vi "Hardware - XNET CAN Host.vi"() -> ()   [LabVIEW 2015, in "ECS-Host.lvlib"]
uses:
  ECS-Host.lvlib
  Typedefs/MISC/Control Parameters.ctl
  ECS-Shared.lvlib
panel:
  out "Loop Duration":u32 caption="[ms]"
  in  "Loop Period":u32 caption="[ms]"
  in  "Refresh Database":bool
  out "CAN Tx Signals":sgl[](array[numeric])
  out "Tx Data":sgl[](array[numeric]) caption="data" format="%.2f"
  in  "Tx Signals":string
  in  "_Tx Signals Mem":string[](array[string])
  in  "CalPointIDs":sgl[](array[numeric])
  out "NamesShort":string
  out "CAN Rx Signals":sgl[](array[numeric])
  in  "Rx Signals":string
  out "Rx Data":sgl[](array[numeric]) caption="data" format="%.2f"
  in  "_Rx Signals Mem":string[](array[string])
  in  "ControlParamMem":string
  in  "_Control Param Array":T1[](array[typedef])
  out "XNET_Fault":bool
  in  "_Refresh (Hidden)":bool
  out "DatabaseAlias":string
  out "CAN Interfaces":sgl[](array[numeric])
  out "IP_Address":string="0.0.0.0"
  in  "CAN Interface":u8
  out "CAN ECUs":sgl[](array[numeric])
  out "CAN Clusters":sgl[](array[numeric])
  out "XNET_Fault_Code":i32
  out "XNET_Fault_Desc":string
  in  "_CalPoints Select":u32(ring) caption="CalPoints Select"
  out "_XNET Error":T2 caption="XNET Error"
  in  "Deployed ECUs":i32(listbox) caption="Deployed Databases"
  in  "Deployed Clusters":i32(listbox) caption="Deployed Databases"
  in  "Intf_CAN_Term":bool caption="Termination"
  in  "Baud_Rate":u32 caption="Baud Rate"
  in  "Deployed Databases":i32(listbox)
  in  "CAN_Run":bool
  in  "_CAN Tx Signal":u16(ring) caption="CAN Signal" items=["Not Selected"]
  in  "_Tx.Insert":bool
  in  "_Tx.Up":bool
  in  "_Tx.Delete":bool
  in  "_Tx.Down":bool
  in  "_Tx Table":i32(listbox)
  in  "_CAN Rx Signal":u16(ring) caption="CAN Signal" items=["Not Selected"]
  in  "_Rx.Insert":bool
  in  "_Rx.Up":bool
  in  "_Rx.Delete":bool
  in  "_Rx.Down":bool
  in  "_CAN Interface":u8(ring) caption="CAN Interface"
  in  "_Control Parameter":T1=enum."Pedal Position [%]" caption="Control Parameters"
  in  "_Rx Table":i32(listbox)
  # "---- Rx ---->"
  # "READ FROM\nCAN BUS"
  # "-------- Tx -------->"
  # "WRITE TO\nCAN BUS"
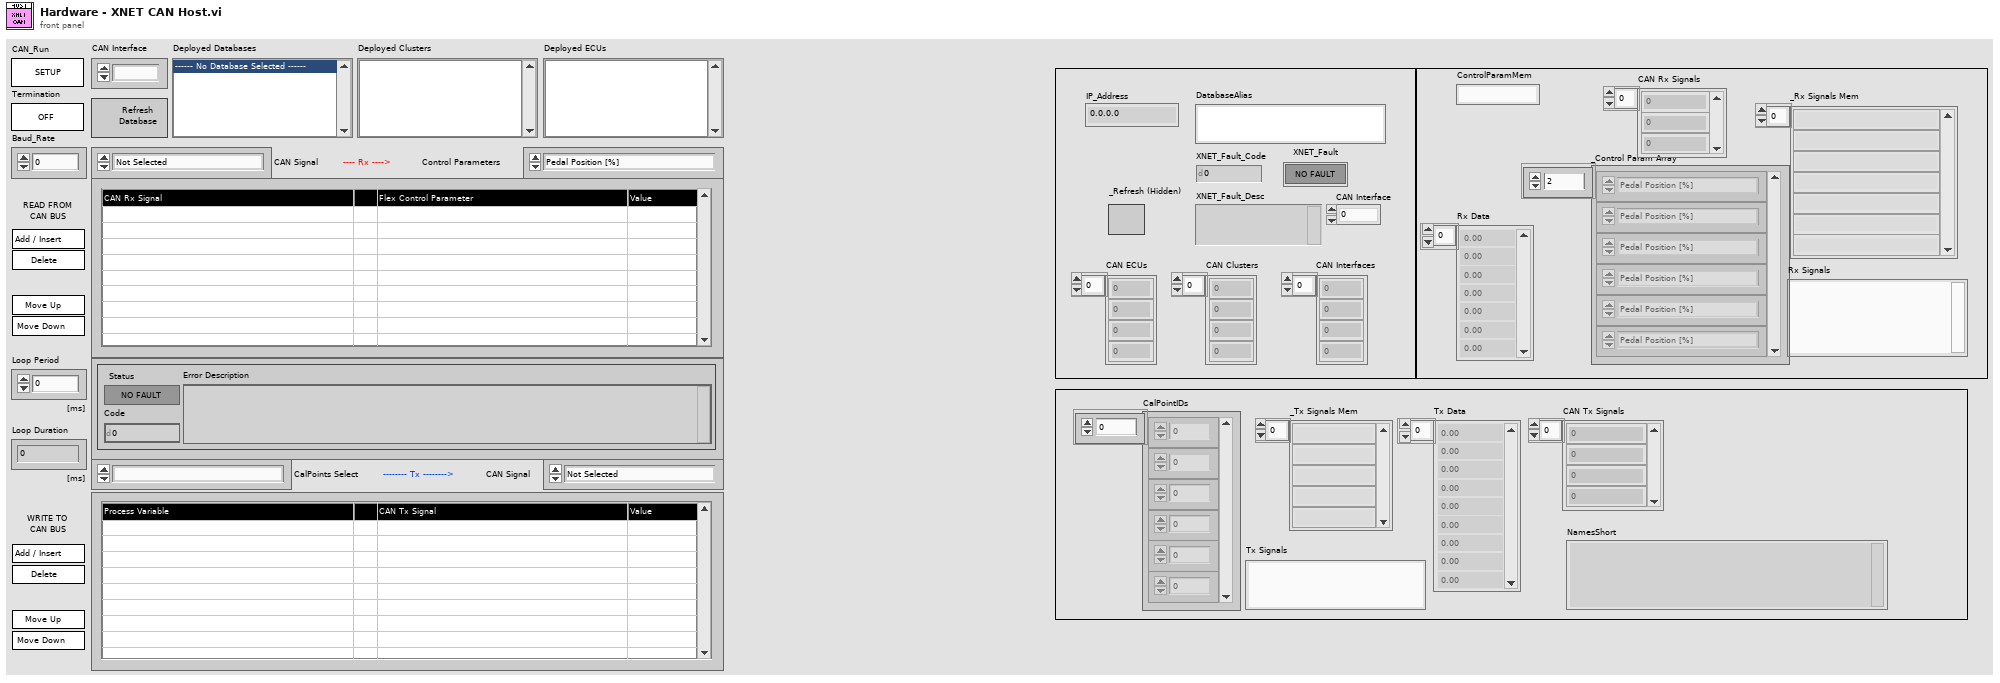
[diagram p1: front panel]
types:
  T1 = typedef "ECS-Shared.lvlib/Control Parameters.ctl" = enum16{"Not Selected", "Pedal Position [%]", "ESTOP", "Sensor1NOx", "Sensor1O2", "Sensor1SupplyStatus", "Sensor1TempStatus", "Sensor1NOxStatus", "Sensor1O2Status", "Sensor1HeaterMode", "Sensor1HeaterCircuit", "Sensor1NOxCircuit", "Sensor1O2Circuit", "Sensor2NOx", "Sensor2O2", "Sensor2SupplyStatus", "Sensor2TempStatus", "Sensor2NOxStatus", "Sensor2O2Status", "Sensor2HeaterMode", "Sensor2HeaterCircuit", "Sensor2NOxCircuit", "Sensor2O2Circuit"}
  T2 = cluster{"Status":bool, "Code":i32, "Error Description":string}
  T3 = enum8{"Enabled", "Disabled", "Disabled and Grayed Out"}
  T4 = cluster{"Status":bool, "Code":i32, "Desc":string}
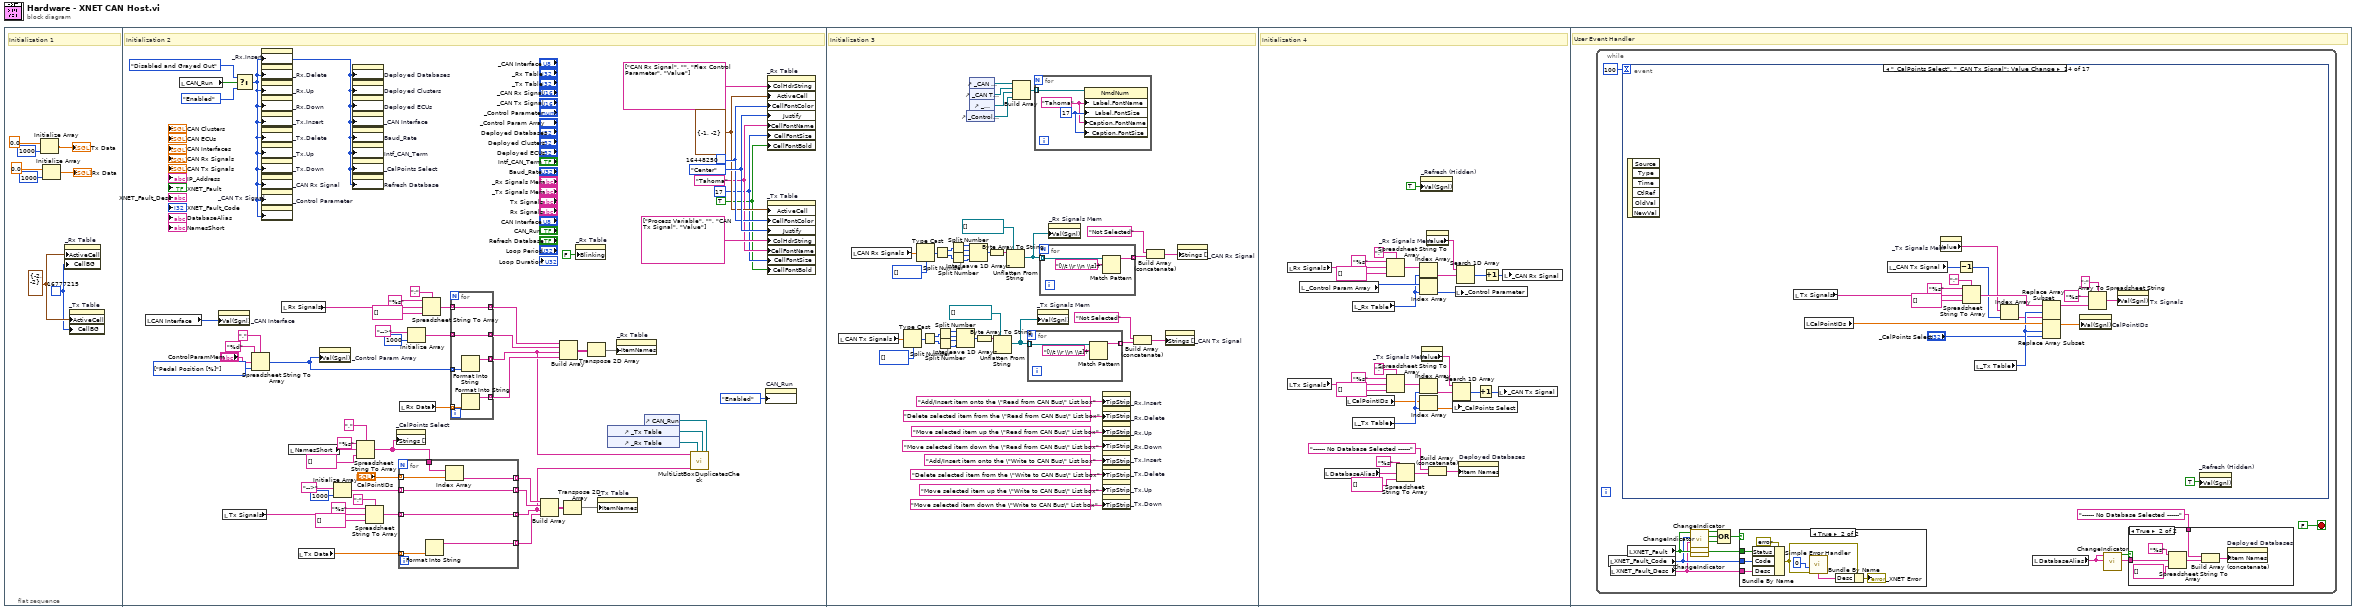
[diagram p0: block diagram]
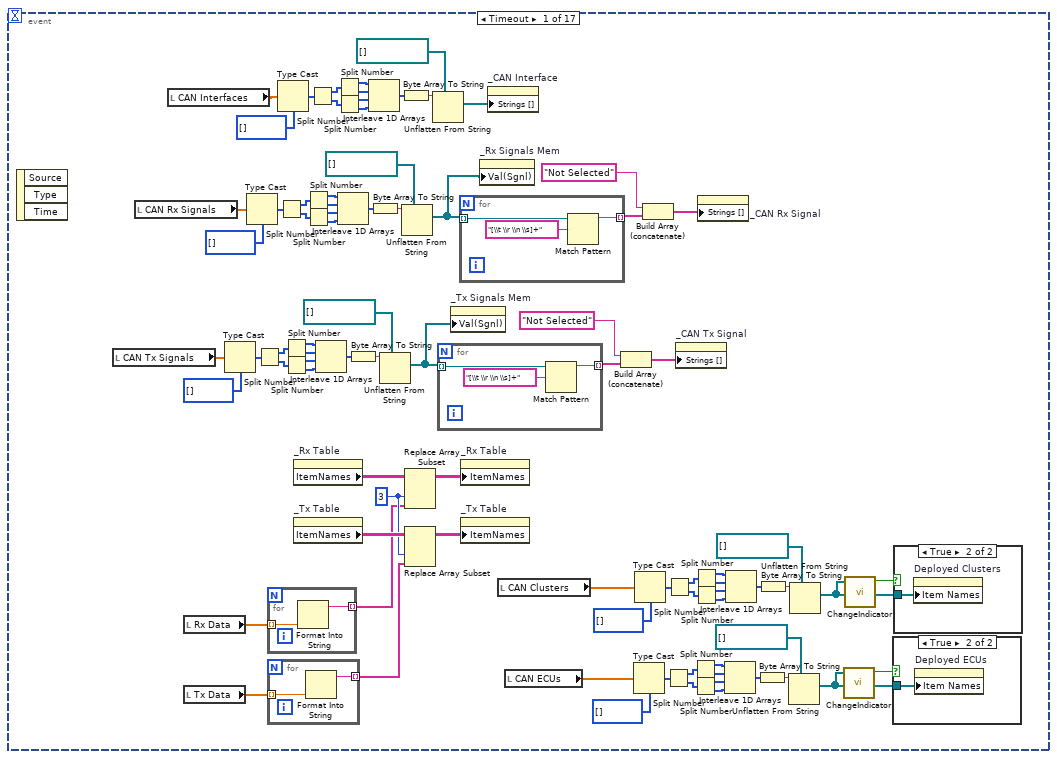
[diagram p4: hidden frame]
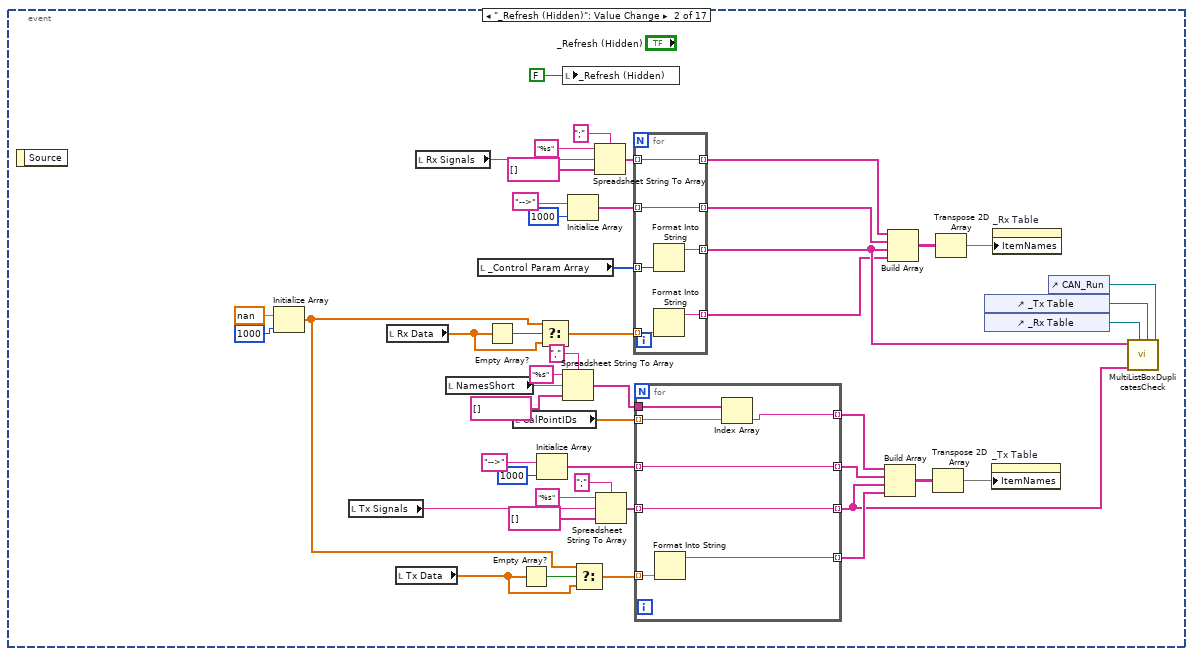
[diagram p7: hidden frame]
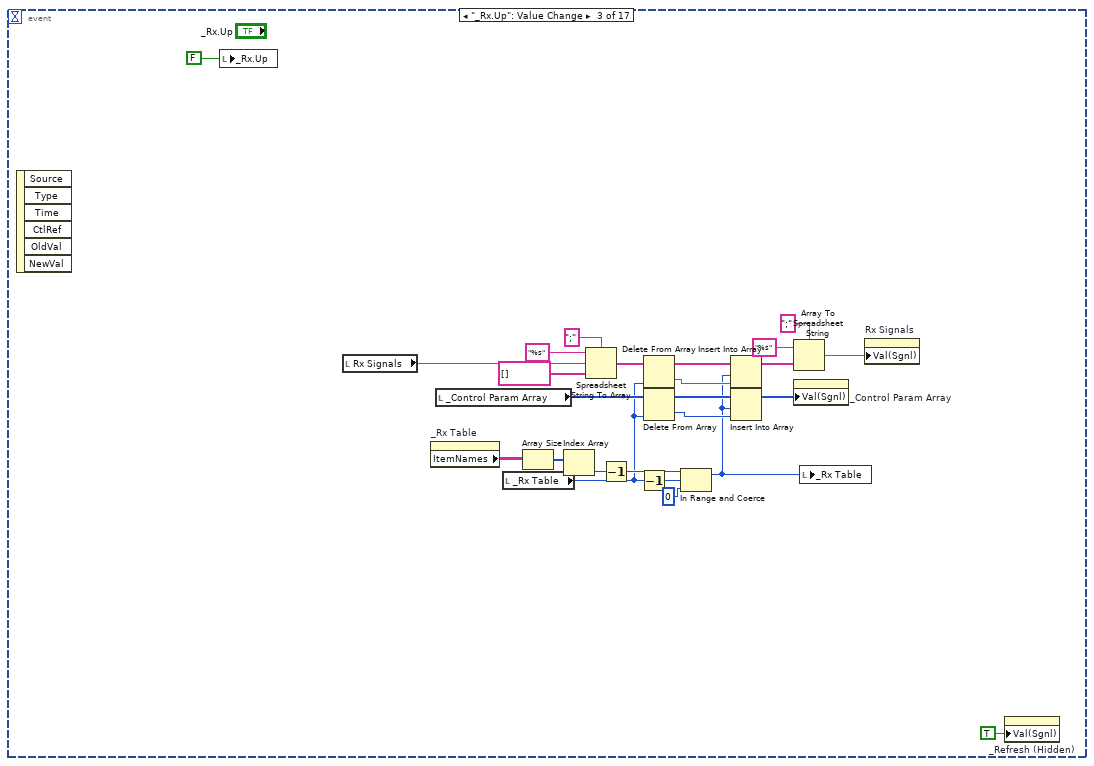
[diagram p8: hidden frame]
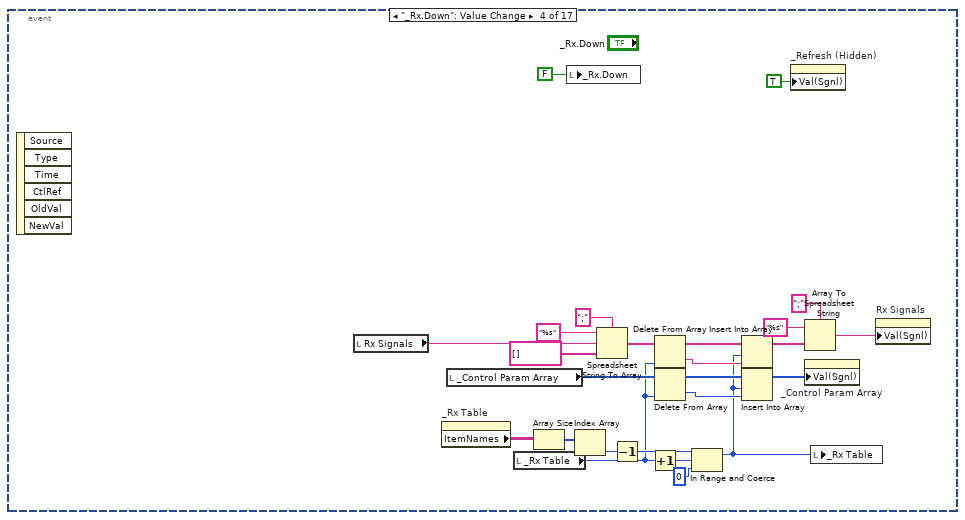
[diagram p9: hidden frame]
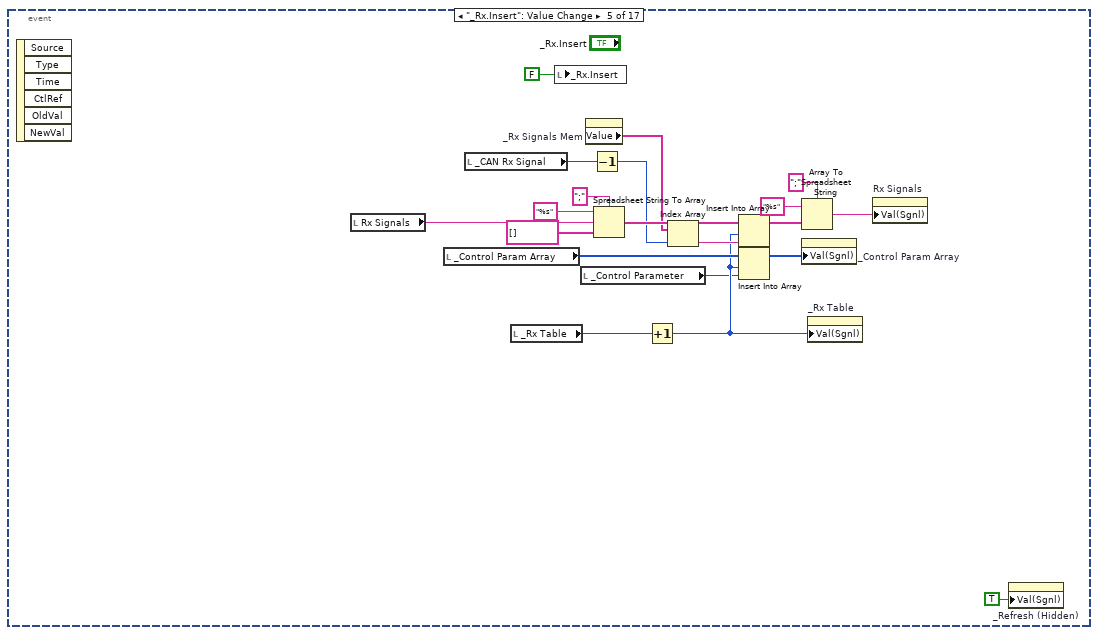
[diagram p10: hidden frame]
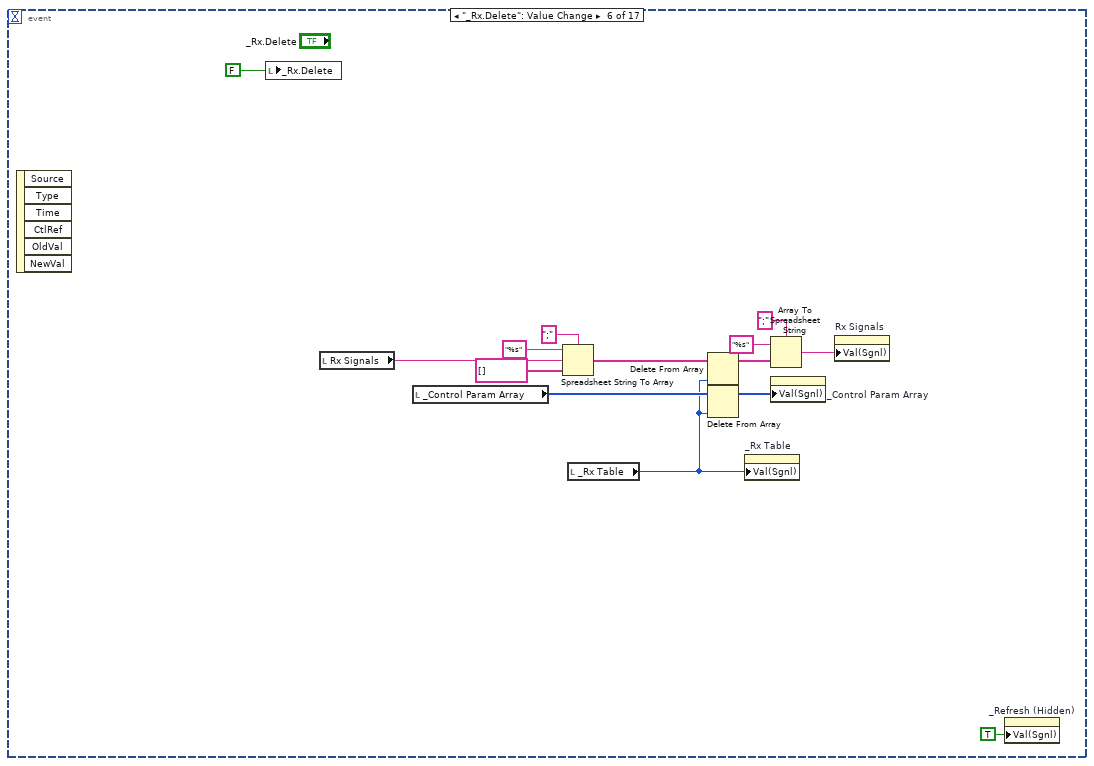
[diagram p11: hidden frame]
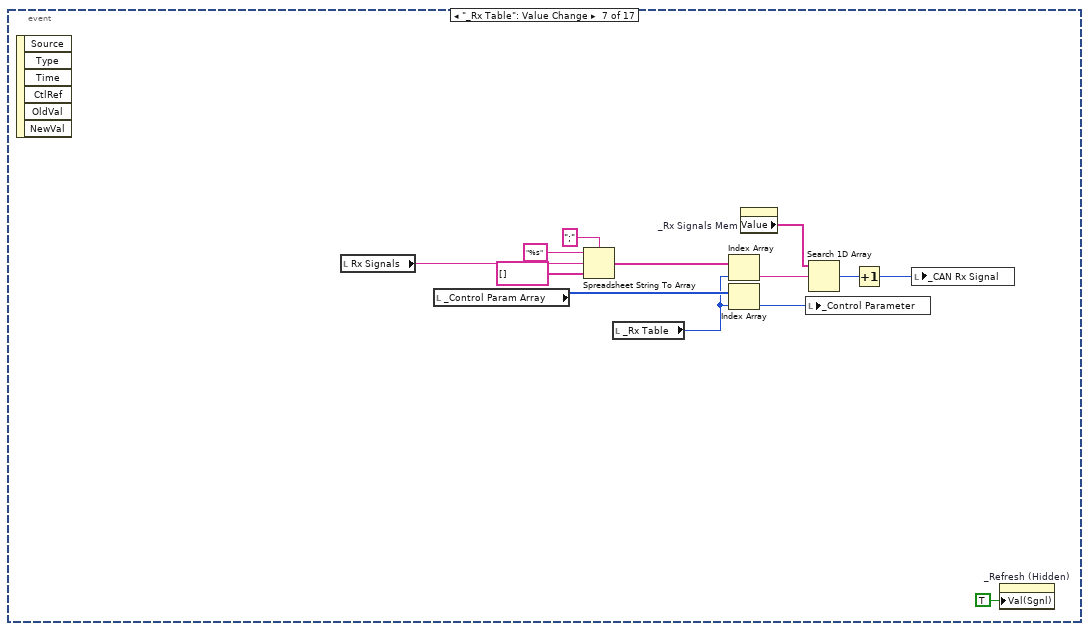
[diagram p12: hidden frame]
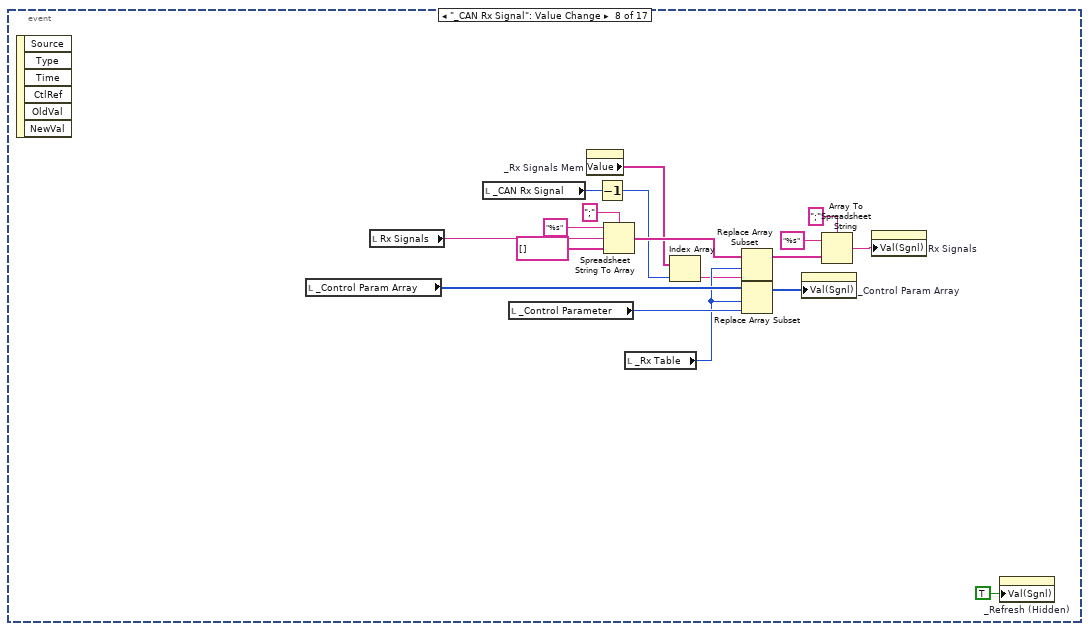
[diagram p13: hidden frame]
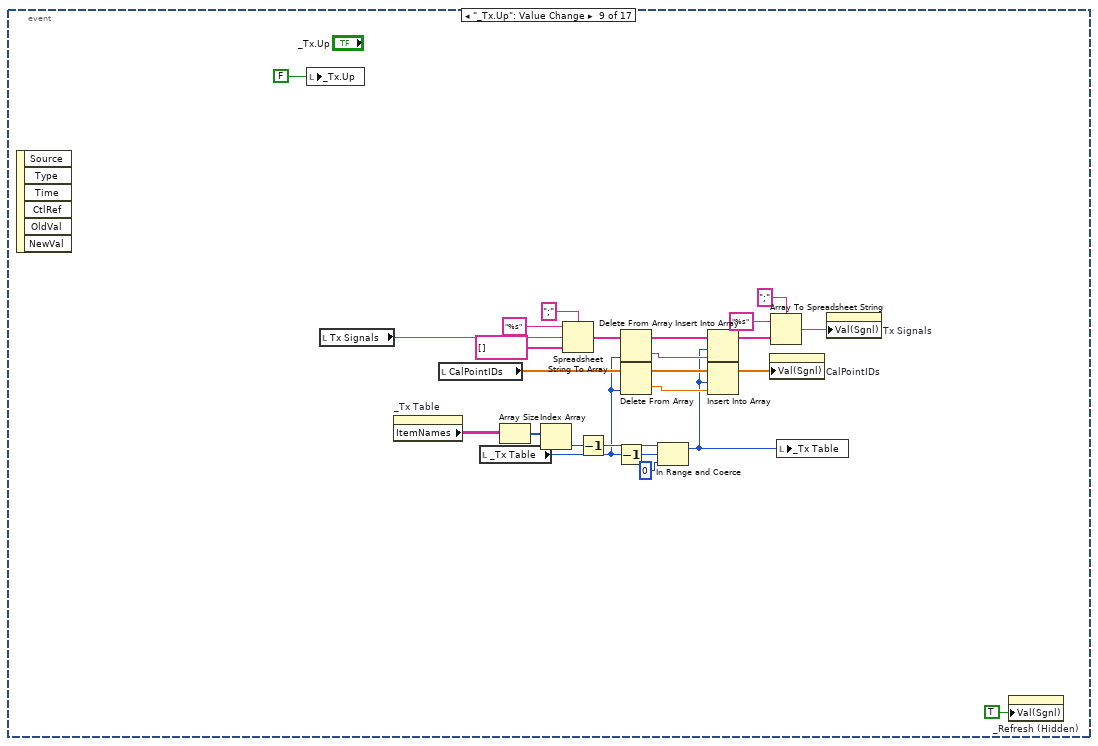
[diagram p14: hidden frame]
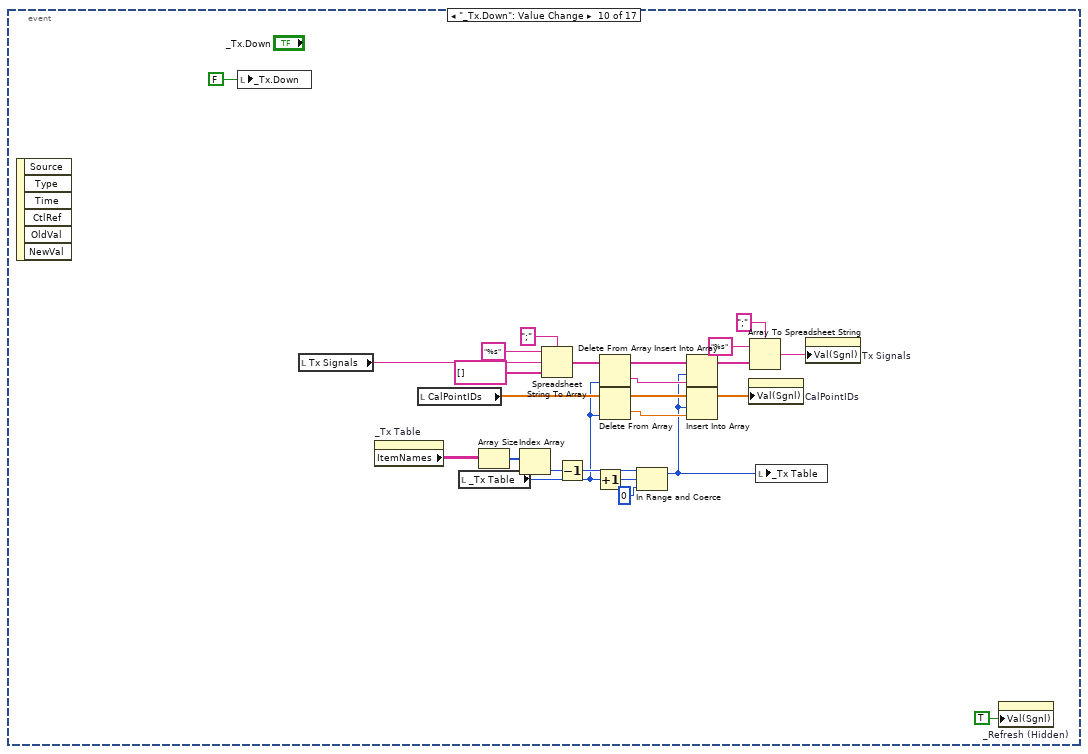
[diagram p15: hidden frame]
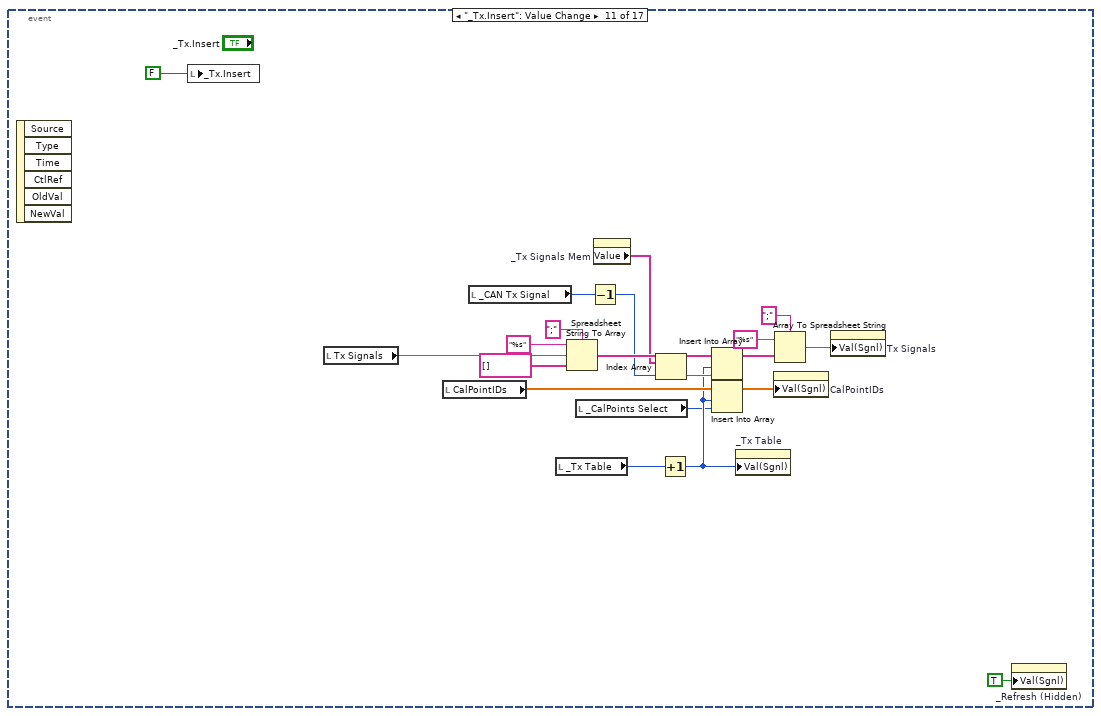
[diagram p16: hidden frame]
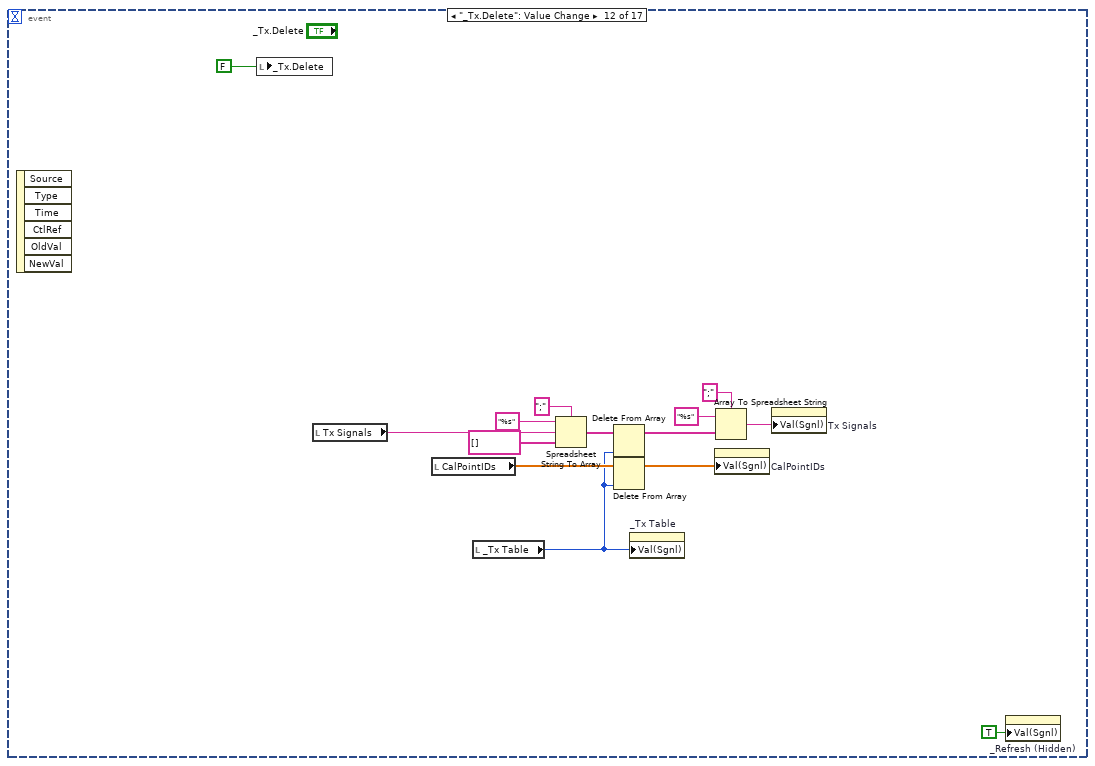
[diagram p17: hidden frame]
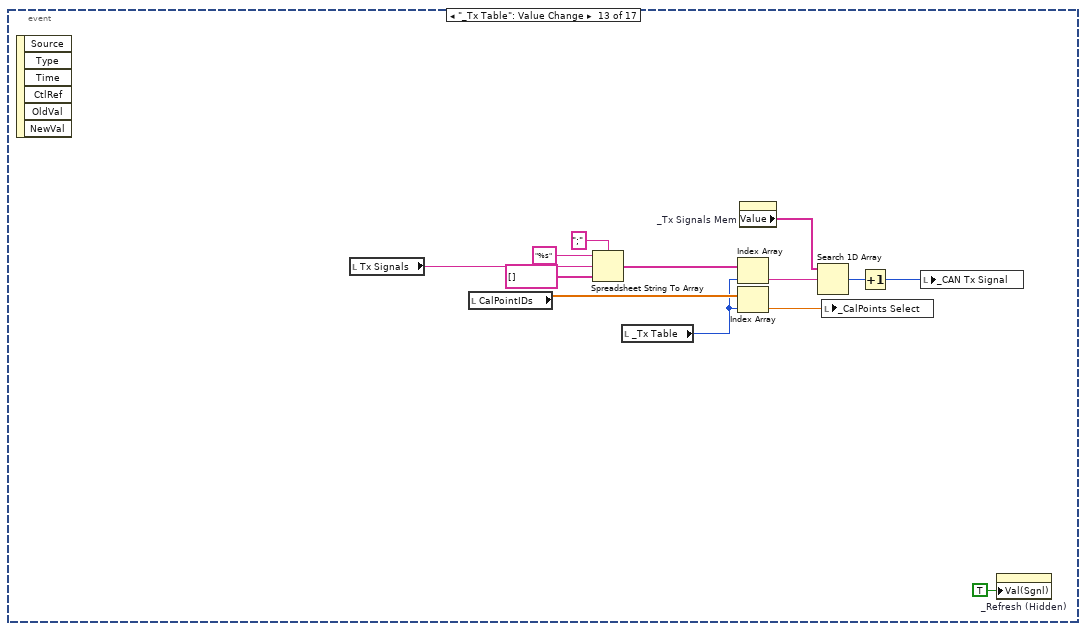
[diagram p18: hidden frame]
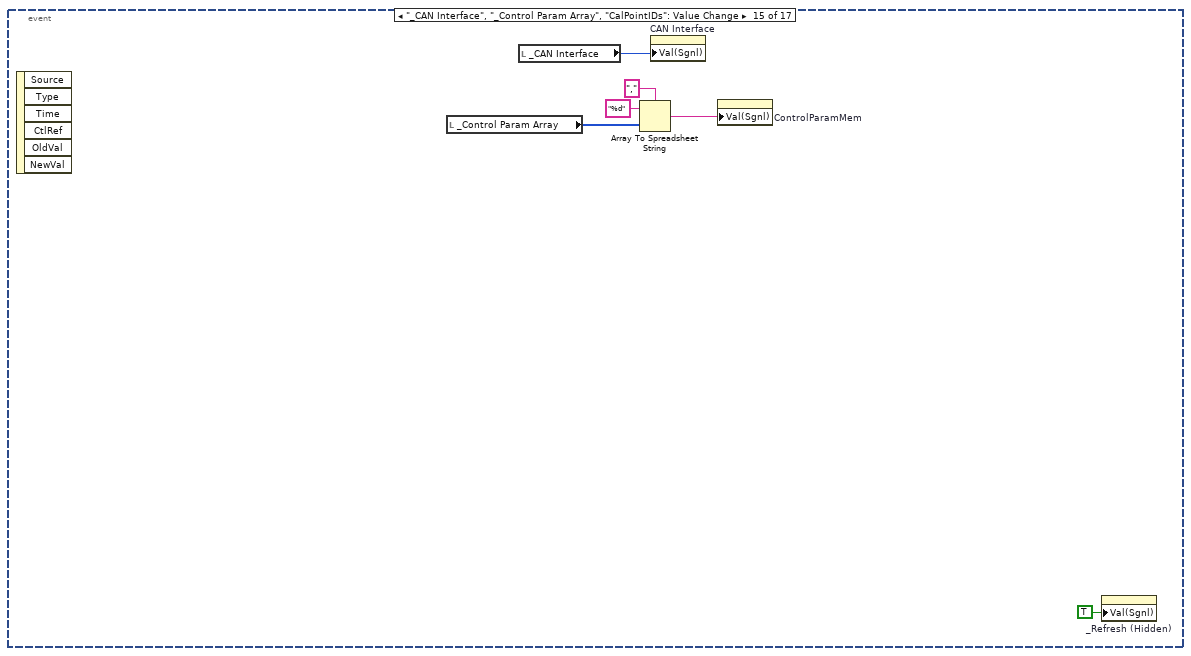
[diagram p19: hidden frame]
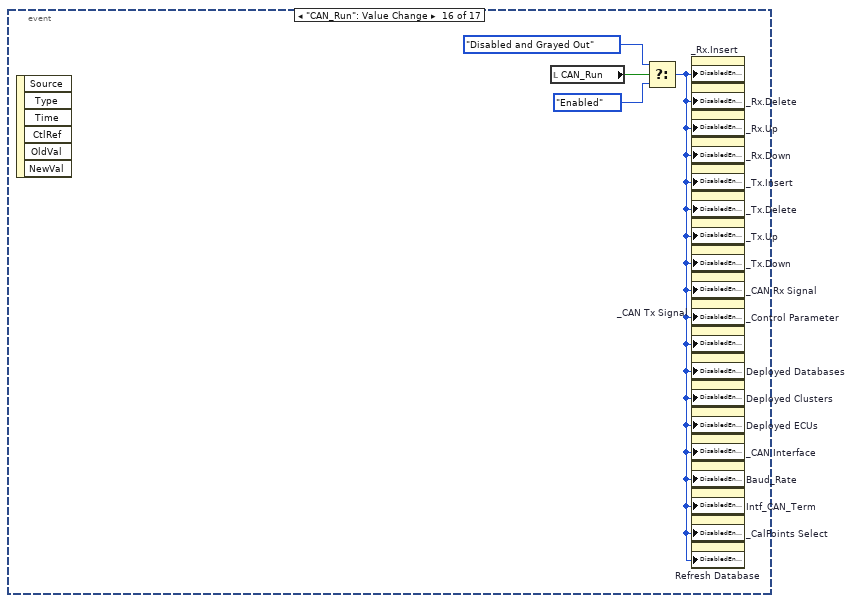
[diagram p20: hidden frame]
diagram:
  n1 = flat-sequence {
    frame #0 {
      w8 = cluster{"Row":i32, "Column":i32} {"Row"=-2, "Column"=-2} ("Active Cell:Active Cell")
      w7 = u32 16777215 ("Color Box")
      # "Initialization 1"
      n2 = Initialize Array(0.0, 1000 ("dimension size")) -> (→"Tx Data":dbl[])
      n3 = Initialize Array(0.0, 1000 ("dimension size")) -> (→"Rx Data":dbl[])
      n4 = property on="_Rx Table" class="MCListbox (strict)"("ActiveCell"=w8, "CellBG"=w7) -> ()  [unwired: 2 in, 2 out]
      n5 = property on="_Tx Table" class="MCListbox (strict)"("ActiveCell"=w8, "CellBG"=w7) -> ()  [unwired: 2 in, 2 out]
    }
    frame #1 {
      w24 = TRUE ("Active Cell:Cell Font:Bold")
      w25 = u32 17 ("Active Cell:Cell Font:Size")
      w26 = "Tahoma" ("Active Cell:Cell Font:Name")
      w29 = enum16{"Left", "Center", "Right"}."Center" ("Active Cell:Cell Justification")
      w28 = u32 16448250
      w27 = cluster{"Row":i32, "Column":i32} {"Row"=-1, "Column"=-2} ("Active Cell:Active Cell")
      w33 = T1[] [enum."Pedal Position [%]"] items=["Not Selected", "Pedal Position [%]", "ESTOP", "Sensor1NOx", "Sensor1O2", "Sensor1SupplyStatus", "Sensor1TempStatus", "Sensor1NOxStatus", "Sensor1O2Status", "Sensor1HeaterMode", "Sensor1HeaterCircuit", "Sensor1NOxCircuit", "Sensor1O2Circuit", "Sensor2NOx", "Sensor2O2", "Sensor2SupplyStatus", "Sensor2TempStatus", "Sensor2NOxStatus", "Sensor2O2Status", "Sensor2HeaterMode", "Sensor2HeaterCircuit", "Sensor2NOxCircuit", "Sensor2O2Circuit"]
      # "Initialization 2"
      n6 = local read "CAN Interface"() -> (w38:u8)
      n7 = local read "CAN_Run"() -> (w35:bool)
      n8 = property on="_CAN Interface" class="Ring (strict)"("Val(Sgnl)"=w38) -> ()  [unwired: 2 in, 2 out]
      n9 = local read "Tx Signals"() -> (w65:string)
      n10 = Select(t=T3."Disabled and Grayed Out" ("Disabled"), s=w35, f=T3."Enabled" ("Disabled")) -> (s? t:f=w9:T3)
      n11 = Spreadsheet String To Array(delimiter (Tab)=",", format string="%d", spreadsheet string="ControlParamMem", array type (2D Dbl)=w33) -> (array=w31:T1[])
      n12 = property on="_Rx.Insert" class="Bool (strict)"("DisabledEnum"=w9) -> ()  [unwired: 2 in, 2 out]
      n13 = property on="_Rx.Delete" class="Bool (strict)"("DisabledEnum"=w9) -> ()  [unwired: 2 in, 2 out]
      n14 = property on="_Rx.Up" class="Bool (strict)"("DisabledEnum"=w9) -> ()  [unwired: 2 in, 2 out]
      n15 = property on="_Rx.Down" class="Bool (strict)"("DisabledEnum"=w9) -> ()  [unwired: 2 in, 2 out]
      n16 = property on="_Tx.Insert" class="Bool (strict)"("DisabledEnum"=w9) -> ()  [unwired: 2 in, 2 out]
      n17 = property on="_Tx.Delete" class="Bool (strict)"("DisabledEnum"=w9) -> ()  [unwired: 2 in, 2 out]
      n18 = property on="_Tx.Up" class="Bool (strict)"("DisabledEnum"=w9) -> ()  [unwired: 2 in, 2 out]
      n19 = property on="_Tx.Down" class="Bool (strict)"("DisabledEnum"=w9) -> ()  [unwired: 2 in, 2 out]
      n20 = property on="_CAN Rx Signal" class="Ring (strict)"("DisabledEnum"=w9) -> ()  [unwired: 2 in, 2 out]
      n21 = property on="_CAN Tx Signal" class="Ring (strict)"("DisabledEnum"=w9) -> ()  [unwired: 2 in, 2 out]
      n22 = property on="_Control Parameter" class="Enum (strict)"("DisabledEnum"=w9) -> ()  [unwired: 2 in, 2 out]
      n23 = local read "Rx Signals"() -> (w61:string)
      n24 = local read "NamesShort"() -> (w15:string)
      n25 = local read "Tx Data"() -> (w52:sgl[])
      n26 = property on="_Control Param Array" class="Arr (strict)"("Val(Sgnl)"=w31) -> ()  [unwired: 2 in, 2 out]
      n27 = Initialize Array("-->", 1000 ("dimension size")) -> (w50:string[])
      n28 = property on="Deployed Databases" class="LstBox (strict)"("DisabledEnum"=w9) -> ()  [unwired: 2 in, 2 out]
      n29 = property on="Deployed Clusters" class="LstBox (strict)"("DisabledEnum"=w9) -> ()  [unwired: 2 in, 2 out]
      n30 = property on="Deployed ECUs" class="LstBox (strict)"("DisabledEnum"=w9) -> ()  [unwired: 2 in, 2 out]
      n31 = property on="_CAN Interface" class="Ring (strict)"("DisabledEnum"=w9) -> ()  [unwired: 2 in, 2 out]
      n32 = property on="Baud_Rate" class="DigNum (strict)"("DisabledEnum"=w9) -> ()  [unwired: 2 in, 2 out]
      n33 = property on="Intf_CAN_Term" class="Bool (strict)"("DisabledEnum"=w9) -> ()  [unwired: 2 in, 2 out]
      n34 = property on="_CalPoints Select" class="Ring (strict)"("DisabledEnum"=w9) -> ()  [unwired: 2 in, 2 out]
      n35 = property on="Refresh Database" class="Bool (strict)"("DisabledEnum"=w9) -> ()  [unwired: 2 in, 2 out]
      n36 = Spreadsheet String To Array(delimiter (Tab)=",", format string="%s", spreadsheet string=w15, array type (2D Dbl)=string[] []) -> (array=w12:string[])
      n37 = Spreadsheet String To Array(delimiter (Tab)=";", format string="%s", spreadsheet string=w65, array type (2D Dbl)=string[] []) -> (array=w39:string[])
      n38 = property on="_CalPoints Select" class="Ring (strict)"("Strings []"=w12) -> ()  [unwired: 2 in, 2 out]
      n39 = for {
        tunnel: w52 -> [w73] mode=indexing
        tunnel: w50 -> [w74] mode=indexing
        tunnel: [w68] -> w54 mode=indexing
        tunnel: [w74] -> w53 mode=indexing
        tunnel: [w71] -> w19 mode=indexing
        tunnel: [w72] -> w49 mode=indexing
        tunnel: w39 -> [w71] mode=indexing
        tunnel: "CalPointIDs" -> [w70] mode=indexing
        tunnel: w12 -> [w69]
        n40 = Format Into String(w73) -> (resulting string=w72:string)  [unwired: 3 in, 1 out]
        n41 = Index Array(array=w69, index=w70) -> (element=w68:string)
      }
      n42 = local read "Rx Data"() -> (w44:sgl[])
      n43 = Initialize Array("-->", 1000 ("dimension size")) -> (w47:string[])
      n44 = Spreadsheet String To Array(delimiter (Tab)=";", format string="%s", spreadsheet string=w61, array type (2D Dbl)=string[] []) -> (array=w60:string[])
      n45 = for {
        tunnel: w60 -> [w78] mode=indexing
        tunnel: w31 -> [w75] mode=indexing
        tunnel: w44 -> [w80] mode=indexing
        tunnel: w47 -> [w79] mode=indexing
        tunnel: [w78] -> w40 mode=indexing
        tunnel: [w79] -> w41 mode=indexing
        tunnel: [w77] -> w18 mode=indexing
        tunnel: [w76] -> w48 mode=indexing
        n46 = Format Into String(w75) -> (resulting string=w77:string)  [unwired: 3 in, 1 out]
        n47 = Format Into String(w80) -> (resulting string=w76:string)  [unwired: 3 in, 1 out]
      }
      n48 = Build Array(w54, w53, w19, w49) -> (w11:string[][])
      n49 = Build Array(w40, w41, w18, w48) -> (w42:string[][])
      n50 = Transpose 2D Array(2D array=w11) -> (transposed array=w56:string[][])
      n51 = property on="_Rx Table" class="MCListbox (strict)"("Blinking"=FALSE) -> ()  [unwired: 2 in, 2 out]
      n52 = Transpose 2D Array(2D array=w42) -> (transposed array=w43:string[][])
      n53 = property on="_Tx Table" class="MCListbox (strict)"("ItemNames"=w56) -> ()  [unwired: 2 in, 2 out]
      n54 = control-ref of="_Tx Table"() -> (w21:refnum<vi>)
      n55 = control-ref of="_Rx Table"() -> (w20:refnum<vi>)
      n56 = property on="_Rx Table" class="MCListbox (strict)"("ItemNames"=w43) -> ()  [unwired: 2 in, 2 out]
      n57 = control-ref of="CAN_Run"() -> (w22:refnum<vi>)
      n58 = call "MultiListBoxDuplicatesCheck.vi"("CAN Init Ref In"=w22, "_Write Table In"=w21, "_Read Table Ref In"=w20, "CAN Write Signals String Array"=w19, "Flex Control Parameters String Array"=w18) -> ()  [unwired: 7 in]
      n59 = property on="CAN_Run" class="Bool (strict)"("DisabledEnum"=T3."Enabled" ("Disabled")) -> ()  [unwired: 2 in, 2 out]
      n60 = property on="_Rx Table" class="MCListbox (strict)"("ColHdrString"=string[] ["CAN Rx Signal", "", "Flex Control Parameter", "Value"] ("Column Header Strings[]"), "ActiveCell"=w27, "CellFontColor"=w28, "Justify"=w29, "CellFontName"=w26, "CellFontSize"=w25, "CellFontBold"=w24) -> ()  [unwired: 2 in, 2 out]
      n61 = property on="_Tx Table" class="MCListbox (strict)"("ActiveCell"=w27, "CellFontColor"=w28, "Justify"=w29, "ColHdrString"=string[] ["Process Variable", "", "CAN Tx Signal", "Value"] ("Column Header Strings[]"), "CellFontName"=w26, "CellFontSize"=w25, "CellFontBold"=w24) -> ()  [unwired: 2 in, 2 out]
    }
    frame #2 {
      # "Initialization 3"
      n62 = local read "CAN Tx Signals"() -> (w113:sgl[])
      n63 = local read "CAN Rx Signals"() -> (w105:sgl[])
      n64 = Type Cast(type=u32[] [], x=w113) -> (*(type *) &x=w115:u32[])
      n65 = Type Cast(type=u32[] [], x=w105) -> (*(type *) &x=w103:u32[])
      n66 = Split Number(x=w115) -> (hi(x)=w117:u16[], lo(x)=w116:u16[])
      n67 = Split Number(x=w103) -> (hi(x)=w101:u16[], lo(x)=w102:u16[])
      n68 = Split Number(x=w117) -> (hi(x)=w118:u8[], lo(x)=w119:u8[])
      n69 = Split Number(x=w116) -> (hi(x)=w120:u8[], lo(x)=w121:u8[])
      n70 = Split Number(x=w101) -> (hi(x)=w100:u8[], lo(x)=w99:u8[])
      n71 = Split Number(x=w102) -> (hi(x)=w98:u8[], lo(x)=w97:u8[])
      n72 = Interleave 1D Arrays(w118, w119, w120, w121) -> (w122:u8[])
      n73 = control-ref of="_Control Parameter"() -> (w87:refnum<vi>)
      n74 = Interleave 1D Arrays(w100, w99, w98, w97) -> (w96:u8[])
      n75 = control-ref of="_CAN Rx Signal"() -> (w89:refnum<vi>)
      n76 = control-ref of="_CAN Tx Signal"() -> (w88:refnum<vi>)
      n77 = control-ref of="_CalPoints Select"() -> (w81:refnum<vi>)
      n78 = Byte Array To String(unsigned byte array=w122) -> (string=w123:string)
      n79 = Byte Array To String(unsigned byte array=w96) -> (string=w95:string)
      n80 = Unflatten From String(type=refnum<k21>[] [] ("Devices"), binary string=w123) -> (value=w125:refnum<k21>[])  [unwired: 3 in, 2 out]
      n81 = Unflatten From String(type=refnum<k21>[] [] ("Devices"), binary string=w95) -> (value=w106:refnum<k21>[])  [unwired: 3 in, 2 out]
      n82 = Build Array(w89, w88, w81, w87) -> (w86:refnum<vi>[])
      n83 = for {
        tunnel: [w131] -> w112 mode=indexing
        tunnel: w125 -> [w130] mode=indexing
        n84 = Match Pattern(string=w130, regular expression="[\\t \\r \\n \\s]+") -> (before substring=w131:string)  [unwired: 1 in, 3 out]
      }
      n85 = for {
        tunnel: w86 -> [w128] mode=indexing
        w126 = "Tahoma" ("Label.Font:Name")
        w127 = u32 17 ("Label.Font:Size")
        n86 = property class="NmdNum"(reference=w128, "Label.FontName"=w126, "Label.FontSize"=w127, "Caption.FontName"=w126, "Caption.FontSize"=w127) -> ()  [unwired: 1 in, 2 out]
      }
      n87 = property on="_Tx Signals Mem" class="Arr (strict)"("Val(Sgnl)"=w125) -> ()  [unwired: 2 in, 2 out]
      n88 = for {
        tunnel: [w134] -> w107 mode=indexing
        tunnel: w106 -> [w133] mode=indexing
        n89 = Match Pattern(string=w133, regular expression="[\\t \\r \\n \\s]+") -> (before substring=w134:string)  [unwired: 1 in, 3 out]
      }
      n90 = property on="_Rx Signals Mem" class="Arr (strict)"("Val(Sgnl)"=w106) -> ()  [unwired: 2 in, 2 out]
      n91 = property on="_Rx.Insert" class="Bool (strict)"("TipStrip"="Add/Insert item onto the \"Read from CAN Bus\" List box" ("Label.Font:Name")) -> ()  [unwired: 2 in, 2 out]
      n92 = property on="_Rx.Delete" class="Bool (strict)"("TipStrip"="Delete selected item from the \"Read from CAN Bus\" List box" ("Label.Font:Name")) -> ()  [unwired: 2 in, 2 out]
      n93 = property on="_Rx.Up" class="Bool (strict)"("TipStrip"="Move selected item up the \"Read from CAN Bus\" List box" ("Label.Font:Name")) -> ()  [unwired: 2 in, 2 out]
      n94 = property on="_Rx.Down" class="Bool (strict)"("TipStrip"="Move selected item down the \"Read from CAN Bus\" List box" ("Label.Font:Name")) -> ()  [unwired: 2 in, 2 out]
      n95 = property on="_Tx.Insert" class="Bool (strict)"("TipStrip"="Add/Insert item onto the \"Write to CAN Bus\" List box" ("Label.Font:Name")) -> ()  [unwired: 2 in, 2 out]
      n96 = property on="_Tx.Delete" class="Bool (strict)"("TipStrip"="Delete selected item from the \"Write to CAN Bus\" List box" ("Label.Font:Name")) -> ()  [unwired: 2 in, 2 out]
      n97 = property on="_Tx.Up" class="Bool (strict)"("TipStrip"="Move selected item up the \"Write to CAN Bus\" List box" ("Label.Font:Name")) -> ()  [unwired: 2 in, 2 out]
      n98 = property on="_Tx.Down" class="Bool (strict)"("TipStrip"="Move selected item down the \"Write to CAN Bus\" List box" ("Label.Font:Name")) -> ()  [unwired: 2 in, 2 out]
      n99 = Build Array (concatenate)("Not Selected", w112) -> (w110:string[])
      n100 = Build Array (concatenate)("Not Selected", w107) -> (w109:string[])
      n101 = property on="_CAN Tx Signal" class="Ring (strict)"("Strings []"=w110) -> ()  [unwired: 2 in, 2 out]
      n102 = property on="_CAN Rx Signal" class="Ring (strict)"("Strings []"=w109) -> ()  [unwired: 2 in, 2 out]
    }
    frame #3 {
      # "Initialization 4"
      n103 = local read "Rx Signals"() -> (w162:string)
      n104 = local read "Tx Signals"() -> (w150:string)
      n105 = local read "_Control Param Array"() -> (w160:T1[])
      n106 = local read "DatabaseAlias"() -> (w142:string)
      n107 = local read "CalPointIDs"() -> (w136:sgl[])
      n108 = local read "_Rx Table"() -> (w159:i32)
      n109 = local read "_Tx Table"() -> (w148:i32)
      n110 = Spreadsheet String To Array(delimiter (Tab)=";", format string="%s", spreadsheet string=w162, array type (2D Dbl)=string[] []) -> (array=w161:string[])
      n111 = Spreadsheet String To Array(delimiter (Tab)=";", format string="%s", spreadsheet string=w150, array type (2D Dbl)=string[] []) -> (array=w149:string[])
      n112 = Spreadsheet String To Array(format string="%s", spreadsheet string=w142, array type (2D Dbl)=string[] []) -> (array=w139:string[])  [unwired: 1 in]
      n113 = Index Array(array=w161, index=w159) -> (element=w157:string)
      n114 = Index Array(array=w160, index=w159) -> (element=w158:T1)
      n115 = Index Array(array=w149, index=w148) -> (element=w147:string)
      n116 = Index Array(array=w136, index=w148) -> (element=w135:sgl)
      n117 = property on="_Refresh (Hidden)" class="Bool (strict)"("Val(Sgnl)"=TRUE ("Value (Signaling)")) -> ()  [unwired: 2 in, 2 out]
      n118 = property on="_Tx Signals Mem" class="Arr (strict)"() -> ("Value"=w144:string[])  [unwired: 2 in, 2 out]
      n119 = property on="_Rx Signals Mem" class="Arr (strict)"() -> ("Value"=w155:string[])  [unwired: 2 in, 2 out]
      n120 = Build Array (concatenate)("------ No Database Selected ------" ("DatabaseAlias"), w139) -> (w138:string[])
      n121 = Search 1D Array(1D array=w144, element=w147) -> (index of element=w146:i32)  [unwired: 1 in]
      n122 = local write "_CalPoints Select"(w135) -> ()
      n123 = local write "_Control Parameter"(w158) -> ()
      n124 = Search 1D Array(1D array=w155, element=w157) -> (index of element=w156:i32)  [unwired: 1 in]
      n125 = property on="Deployed Databases" class="LstBox (strict)"("Item Names"=w138) -> ()  [unwired: 2 in, 2 out]
      n126 = Increment(x=w146) -> (x+1=w145:i32)
      n127 = Increment(x=w156) -> (x+1=w154:i32)
      n128 = local write "_CAN Tx Signal"(w145) -> ()
      n129 = local write "_CAN Rx Signal"(w154) -> ()
    }
    frame #4 {
      # "User Event Handler"
      n130 = while {
        stop <- FALSE stop-if-true
        n131 = local read "XNET_Fault_Code"() -> (w167:i32)
        n132 = local read "XNET_Fault_Desc"() -> (w166:string)
        n133 = event shown="[13] \"_CalPoints Select\", \"_CAN Tx Signal\": Value Change" {
          selector: _ -> [_ _ _ _ _ _ _ _ _ _ _ _ _ _ _ _ _]
          dyn-events: _ -> [_ _ _ _ _ _ _ _ _ _ _ _ _ _ _ _ _]
          timeout: 100 -> [_ _ _ _ _ _ _ _ _ _ _ _ _ _ _ _ _]
          event Timeout {
            w243 = 3 ("disabled index (col)")
            n134 = event-data() -> ()  [unwired: 1 in, 3 out]
            n135 = local read "CAN Tx Signals"() -> (w236:sgl[])
            n136 = local read "CAN Rx Signals"() -> (w249:sgl[])
            n137 = local read "CAN Interfaces"() -> (w261:sgl[])
            n138 = local read "Rx Data"() -> (w248:sgl[])
            n139 = local read "Tx Data"() -> (w195:sgl[])
            n140 = Type Cast(type=u32[] [], x=w236) -> (*(type *) &x=w234:u32[])
            n141 = Type Cast(type=u32[] [], x=w249) -> (*(type *) &x=w251:u32[])
            n142 = Split Number(x=w234) -> (hi(x)=w232:u16[], lo(x)=w233:u16[])
            n143 = for {
              tunnel: w248 -> [w282] mode=indexing
              tunnel: [w281] -> w242 mode=indexing
              n144 = Format Into String(w282) -> (resulting string=w281:string)  [unwired: 3 in, 1 out]
            }
            n145 = for {
              tunnel: w195 -> [w275] mode=indexing
              tunnel: [w274] -> w194 mode=indexing
              n146 = Format Into String(w275) -> (resulting string=w274:string)  [unwired: 3 in, 1 out]
            }
            n147 = Split Number(x=w251) -> (hi(x)=w253:u16[], lo(x)=w252:u16[])
            n148 = Type Cast(type=u32[] [], x=w261) -> (*(type *) &x=w272:u32[])
            n149 = Split Number(x=w232) -> (hi(x)=w231:u8[], lo(x)=w230:u8[])
            n150 = Split Number(x=w233) -> (hi(x)=w229:u8[], lo(x)=w228:u8[])
            n151 = property on="_Rx Table" class="MCListbox (strict)"() -> ("ItemNames"=w247:string[][])  [unwired: 2 in, 2 out]
            n152 = property on="_Tx Table" class="MCListbox (strict)"() -> ("ItemNames"=w245:string[][])  [unwired: 2 in, 2 out]
            n153 = Split Number(x=w253) -> (hi(x)=w254:u8[], lo(x)=w255:u8[])
            n154 = Split Number(x=w252) -> (hi(x)=w256:u8[], lo(x)=w257:u8[])
            n155 = Split Number(x=w272) -> (hi(x)=w270:u16[], lo(x)=w271:u16[])
            n156 = Interleave 1D Arrays(w231, w230, w229, w228) -> (w227:u8[])
            n157 = Split Number(x=w270) -> (hi(x)=w269:u8[], lo(x)=w268:u8[])
            n158 = Split Number(x=w271) -> (hi(x)=w267:u8[], lo(x)=w266:u8[])
            n159 = Interleave 1D Arrays(w254, w255, w256, w257) -> (w258:u8[])
            n160 = Byte Array To String(unsigned byte array=w227) -> (string=w226:string)
            n161 = Interleave 1D Arrays(w269, w268, w267, w266) -> (w265:u8[])
            n162 = Byte Array To String(unsigned byte array=w258) -> (string=w259:string)
            n163 = Unflatten From String(type=refnum<k21>[] [] ("Devices"), binary string=w226) -> (value=w192:refnum<k21>[])  [unwired: 3 in, 2 out]
            n164 = Byte Array To String(unsigned byte array=w265) -> (string=w264:string)
            n165 = Unflatten From String(type=refnum<k21>[] [] ("Devices"), binary string=w259) -> (value=w193:refnum<k21>[])  [unwired: 3 in, 2 out]
            n166 = Replace Array Subset(array=w247, new element=w242, index (col)=w243) -> (w246:string[][])  [unwired: 1 in]
            n167 = Replace Array Subset(array=w245, new element=w194, index (col)=w243) -> (w244:string[][])  [unwired: 1 in]
            n168 = Unflatten From String(type=refnum<k21>[] [] ("Devices"), binary string=w264) -> (value=w262:refnum<k21>[])  [unwired: 3 in, 2 out]
            n169 = for {
              tunnel: [w280] -> w237 mode=indexing
              tunnel: w192 -> [w279] mode=indexing
              n170 = Match Pattern(string=w279, regular expression="[\\t \\r \\n \\s]+") -> (before substring=w280:string)  [unwired: 1 in, 3 out]
            }
            n171 = property on="_Tx Signals Mem" class="Arr (strict)"("Val(Sgnl)"=w192) -> ()  [unwired: 2 in, 2 out]
            n172 = for {
              tunnel: [w285] -> w241 mode=indexing
              tunnel: w193 -> [w284] mode=indexing
              n173 = Match Pattern(string=w284, regular expression="[\\t \\r \\n \\s]+") -> (before substring=w285:string)  [unwired: 1 in, 3 out]
            }
            n174 = property on="_Rx Table" class="MCListbox (strict)"("ItemNames"=w246) -> ()  [unwired: 2 in, 2 out]
            n175 = property on="_Tx Table" class="MCListbox (strict)"("ItemNames"=w244) -> ()  [unwired: 2 in, 2 out]
            n176 = property on="_Rx Signals Mem" class="Arr (strict)"("Val(Sgnl)"=w193) -> ()  [unwired: 2 in, 2 out]
            n177 = property on="_CAN Interface" class="Ring (strict)"("Strings []"=w262) -> ()  [unwired: 2 in, 2 out]
            n178 = local read "CAN Clusters"() -> (w223:sgl[])
            n179 = local read "CAN ECUs"() -> (w198:sgl[])
            n180 = Build Array (concatenate)("Not Selected", w237) -> (w196:string[])
            n181 = Type Cast(type=u32[] [], x=w198) -> (*(type *) &x=w200:u32[])
            n182 = Type Cast(type=u32[] [], x=w223) -> (*(type *) &x=w221:u32[])
            n183 = Build Array (concatenate)("Not Selected", w241) -> (w239:string[])
            n184 = Split Number(x=w200) -> (hi(x)=w202:u16[], lo(x)=w201:u16[])
            n185 = Split Number(x=w221) -> (hi(x)=w219:u16[], lo(x)=w220:u16[])
            n186 = property on="_CAN Tx Signal" class="Ring (strict)"("Strings []"=w196) -> ()  [unwired: 2 in, 2 out]
            n187 = Split Number(x=w202) -> (hi(x)=w203:u8[], lo(x)=w204:u8[])
            n188 = Split Number(x=w201) -> (hi(x)=w205:u8[], lo(x)=w206:u8[])
            n189 = Split Number(x=w219) -> (hi(x)=w218:u8[], lo(x)=w217:u8[])
            n190 = Split Number(x=w220) -> (hi(x)=w216:u8[], lo(x)=w215:u8[])
            n191 = property on="_CAN Rx Signal" class="Ring (strict)"("Strings []"=w239) -> ()  [unwired: 2 in, 2 out]
            n192 = Interleave 1D Arrays(w203, w204, w205, w206) -> (w207:u8[])
            n193 = Interleave 1D Arrays(w218, w217, w216, w215) -> (w214:u8[])
            n194 = Byte Array To String(unsigned byte array=w207) -> (string=w208:string)
            n195 = Byte Array To String(unsigned byte array=w214) -> (string=w213:string)
            n196 = Unflatten From String(type=refnum<k21>[] [], binary string=w208) -> (value=w209:refnum<k21>[])  [unwired: 3 in, 2 out]
            n197 = Unflatten From String(type=refnum<k21>[] [], binary string=w213) -> (value=w212:refnum<k21>[])  [unwired: 3 in, 2 out]
            n198 = call "ChangeIndicator.vi"("Input"=w209) -> ("Change"=w210:bool)  [unwired: 9 in]
            n199 = call "ChangeIndicator.vi"("Input"=w212) -> ("Change"=w211:bool)  [unwired: 9 in]
            n200 = case shown="True" w210 {
              tunnel: w209 -> [_ w276]
              frame False {
              }
              frame True {
                n201 = property on="Deployed ECUs" class="LstBox (strict)"("Item Names"=w276) -> ()  [unwired: 2 in, 2 out]
              }
            }
            n202 = case shown="True" w211 {
              tunnel: w212 -> [_ w277]
              frame False {
              }
              frame True {
                n203 = property on="Deployed Clusters" class="LstBox (strict)"("Item Names"=w277) -> ()  [unwired: 2 in, 2 out]
              }
            }
          }
          event "_Refresh (Hidden)": Value Change {
            n204 = event-data() -> ()  [unwired: 1 in, 1 out]
            n205 = Initialize Array(nan ("element"), 1000 ("dimension size")) -> (w298:dbl[])
            n206 = local read "Tx Signals"() -> (w308:string)
            n207 = local read "Rx Data"() -> (w305:sgl[])
            n208 = local read "Tx Data"() -> (w299:sgl[])
            n209 = local read "Rx Signals"() -> (w312:string)
            n210 = local read "NamesShort"() -> (w291:string)
            n211 = local read "_Control Param Array"() -> (w297:T1[])
            n212 = Empty Array?(array=w305) -> (empty?=w306:bool)
            n213 = local read "CalPointIDs"() -> (w289:sgl[])
            n214 = Empty Array?(array=w299) -> (empty?=w301:bool)
            n215 = Initialize Array("-->", 1000 ("dimension size")) -> (w322:string[])
            n216 = Select(t=w298, s=w306, f=w305) -> (s? t:f=w304:dbl[])
            n217 = local write "_Refresh (Hidden)"(FALSE ("_Refresh")) -> ()
            n218 = Spreadsheet String To Array(delimiter (Tab)=",", format string="%s", spreadsheet string=w291, array type (2D Dbl)=string[] []) -> (array=w288:string[])
            n219 = Initialize Array("-->", 1000 ("dimension size")) -> (w325:string[])
            n220 = Select(t=w298, s=w301, f=w299) -> (s? t:f=w300:dbl[])
            n221 = Spreadsheet String To Array(delimiter (Tab)=";", format string="%s", spreadsheet string=w312, array type (2D Dbl)=string[] []) -> (array=w313:string[])
            n222 = Spreadsheet String To Array(delimiter (Tab)=";", format string="%s", spreadsheet string=w308, array type (2D Dbl)=string[] []) -> (array=w307:string[])
            n223 = for {
              tunnel: w313 -> [w344] mode=indexing
              tunnel: w304 -> [w343] mode=indexing
              tunnel: w297 -> [w341] mode=indexing
              tunnel: w325 -> [w346] mode=indexing
              tunnel: [w344] -> w331 mode=indexing
              tunnel: [w346] -> w330 mode=indexing
              tunnel: [w345] -> w333 mode=indexing
              tunnel: [w342] -> w324 mode=indexing
              n224 = Format Into String(w341) -> (resulting string=w345:string)  [unwired: 3 in, 1 out]
              n225 = Format Into String(w343) -> (resulting string=w342:string)  [unwired: 3 in, 1 out]
            }
            n226 = for {
              tunnel: w300 -> [w339] mode=indexing
              tunnel: w322 -> [w340] mode=indexing
              tunnel: [w336] -> w296 mode=indexing
              tunnel: [w340] -> w319 mode=indexing
              tunnel: [w337] -> w286 mode=indexing
              tunnel: [w338] -> w323 mode=indexing
              tunnel: w307 -> [w337] mode=indexing
              tunnel: w289 -> [w335] mode=indexing
              tunnel: w288 -> [w334]
              n227 = Format Into String(w339) -> (resulting string=w338:string)  [unwired: 3 in, 1 out]
              n228 = Index Array(array=w334, index=w335) -> (element=w336:string)
            }
            n229 = Build Array(w296, w319, w286, w323) -> (w320:string[][])
            n230 = Build Array(w331, w330, w333, w324) -> (w329:string[][])
            n231 = Transpose 2D Array(2D array=w320) -> (transposed array=w317:string[][])
            n232 = Transpose 2D Array(2D array=w329) -> (transposed array=w328:string[][])
            n233 = control-ref of="_Tx Table"() -> (w294:refnum<vi>)
            n234 = control-ref of="_Rx Table"() -> (w295:refnum<vi>)
            n235 = property on="_Tx Table" class="MCListbox (strict)"("ItemNames"=w317) -> ()  [unwired: 2 in, 2 out]
            n236 = property on="_Rx Table" class="MCListbox (strict)"("ItemNames"=w328) -> ()  [unwired: 2 in, 2 out]
            n237 = control-ref of="CAN_Run"() -> (w293:refnum<vi>)
            n238 = call "MultiListBoxDuplicatesCheck.vi"("CAN Init Ref In"=w293, "_Write Table In"=w294, "_Read Table Ref In"=w295, "CAN Write Signals String Array"=w286, "Flex Control Parameters String Array"=w333) -> ()  [unwired: 7 in]
          }
          event "_Rx.Up": Value Change {
            n239 = event-data() -> ()  [unwired: 1 in, 6 out]
            n240 = local write "_Rx.Up"(FALSE ("_Up")) -> ()
            n241 = local read "Rx Signals"() -> (w355:string)
            n242 = property on="_Rx Table" class="MCListbox (strict)"() -> ("ItemNames"=w364:string[][])  [unwired: 2 in, 2 out]
            n243 = local read "_Control Param Array"() -> (w362:T1[])
            n244 = local read "_Rx Table"() -> (w347:i32)
            n245 = Array Size(array=w364) -> (size(s)=w369:i32[])
            n246 = Index Array(array=w369) -> (element=w370:i32)  [unwired: 1 in]
            n247 = Spreadsheet String To Array(delimiter (Tab)=";", format string="%s", spreadsheet string=w355, array type (2D Dbl)=string[] []) -> (array=w354:string[])
            n248 = Decrement(x=w370) -> (x-1=w367:i32)
            n249 = Decrement(x=w347) -> (x-1=w368:i32)
            n250 = Delete From Array(array=w354, index=w347) -> (deleted portion=w361:string, array with subset deleted=w363:string[])  [unwired: 1 in]
            n251 = Delete From Array(array=w362, index=w347) -> (deleted portion=w360:T1, array with subset deleted=w365:T1[])  [unwired: 1 in]
            n252 = In Range and Coerce(upper limit=w367, x=w368, lower limit=0) -> (coerced(x)=w348:i32)  [unwired: 1 out]
            n253 = Insert Into Array(array=w363, index=w348, new element=w361) -> (w351:string[])
            n254 = Insert Into Array(array=w365, index=w348, new element=w360) -> (w359:T1[])
            n255 = Array To Spreadsheet String(delimiter (Tab)=";", array=w351, 3:"%s" ("format string")) -> (spreadsheet string=w350:string)
            n256 = property on="_Control Param Array" class="Arr (strict)"("Val(Sgnl)"=w359) -> ()  [unwired: 2 in, 2 out]
            n257 = local write "_Rx Table"(w348) -> ()
            n258 = property on="Rx Signals" class="Str"("Val(Sgnl)"=w350) -> ()  [unwired: 2 in, 2 out]
            n259 = property on="_Refresh (Hidden)" class="Bool (strict)"("Val(Sgnl)"=TRUE ("Value (Signaling)")) -> ()  [unwired: 2 in, 2 out]
          }
          event "_Rx.Down": Value Change {
            n260 = event-data() -> ()  [unwired: 1 in, 6 out]
            n261 = local read "Rx Signals"() -> (w380:string)
            n262 = property on="_Rx Table" class="MCListbox (strict)"() -> ("ItemNames"=w389:string[][])  [unwired: 2 in, 2 out]
            n263 = local read "_Control Param Array"() -> (w387:T1[])
            n264 = local read "_Rx Table"() -> (w372:i32)
            n265 = Array Size(array=w389) -> (size(s)=w394:i32[])
            n266 = local write "_Rx.Down"(FALSE ("_Up")) -> ()
            n267 = Index Array(array=w394) -> (element=w395:i32)  [unwired: 1 in]
            n268 = Spreadsheet String To Array(delimiter (Tab)=";", format string="%s", spreadsheet string=w380, array type (2D Dbl)=string[] []) -> (array=w379:string[])
            n269 = Decrement(x=w395) -> (x-1=w392:i32)
            n270 = Increment(x=w372) -> (x+1=w393:i32)
            n271 = Delete From Array(array=w379, index=w372) -> (deleted portion=w386:string, array with subset deleted=w388:string[])  [unwired: 1 in]
            n272 = Delete From Array(array=w387, index=w372) -> (deleted portion=w385:T1, array with subset deleted=w390:T1[])  [unwired: 1 in]
            n273 = In Range and Coerce(upper limit=w392, x=w393, lower limit=0) -> (coerced(x)=w373:i32)  [unwired: 1 out]
            n274 = Insert Into Array(array=w388, index=w373, new element=w386) -> (w376:string[])
            n275 = Insert Into Array(array=w390, index=w373, new element=w385) -> (w384:T1[])
            n276 = property on="_Refresh (Hidden)" class="Bool (strict)"("Val(Sgnl)"=TRUE ("Value (Signaling)")) -> ()  [unwired: 2 in, 2 out]
            n277 = Array To Spreadsheet String(delimiter (Tab)=";", array=w376, 3:"%s" ("format string")) -> (spreadsheet string=w375:string)
            n278 = property on="_Control Param Array" class="Arr (strict)"("Val(Sgnl)"=w384) -> ()  [unwired: 2 in, 2 out]
            n279 = local write "_Rx Table"(w373) -> ()
            n280 = property on="Rx Signals" class="Str"("Val(Sgnl)"=w375) -> ()  [unwired: 2 in, 2 out]
          }
          event "_Rx.Insert": Value Change {
            n281 = event-data() -> ()  [unwired: 1 in, 6 out]
            n282 = local read "Rx Signals"() -> (w409:string)
            n283 = local read "_Control Param Array"() -> (w403:T1[])
            n284 = local read "_CAN Rx Signal"() -> (w401:u16)
            n285 = local read "_Rx Table"() -> (w414:i32)
            n286 = local write "_Rx.Insert"(FALSE ("_Up")) -> ()
            n287 = local read "_Control Parameter"() -> (w397:T1)
            n288 = property on="_Rx Signals Mem" class="Arr (strict)"() -> ("Value"=w399:string[])  [unwired: 2 in, 2 out]
            n289 = Decrement(x=w401) -> (x-1=w398:u16)
            n290 = Spreadsheet String To Array(delimiter (Tab)=";", format string="%s", spreadsheet string=w409, array type (2D Dbl)=string[] []) -> (array=w404:string[])
            n291 = Increment(x=w414) -> (x+1=w400:i32)
            n292 = Index Array(array=w399, index=w398) -> (element=w402:string)
            n293 = Insert Into Array(array=w404, index=w400, new element=w402) -> (w406:string[])
            n294 = Insert Into Array(array=w403, index=w400, new element=w397) -> (w413:T1[])
            n295 = Array To Spreadsheet String(delimiter (Tab)=";", array=w406, 3:"%s" ("format string")) -> (spreadsheet string=w405:string)
            n296 = property on="_Control Param Array" class="Arr (strict)"("Val(Sgnl)"=w413) -> ()  [unwired: 2 in, 2 out]
            n297 = property on="_Rx Table" class="MCListbox (strict)"("Val(Sgnl)"=w400) -> ()  [unwired: 2 in, 2 out]
            n298 = property on="Rx Signals" class="Str"("Val(Sgnl)"=w405) -> ()  [unwired: 2 in, 2 out]
            n299 = property on="_Refresh (Hidden)" class="Bool (strict)"("Val(Sgnl)"=TRUE ("Value (Signaling)")) -> ()  [unwired: 2 in, 2 out]
          }
          event "_Rx.Delete": Value Change {
            n300 = event-data() -> ()  [unwired: 1 in, 6 out]
            n301 = local write "_Rx.Delete"(FALSE ("_Up")) -> ()
            n302 = local read "Rx Signals"() -> (w424:string)
            n303 = local read "_Control Param Array"() -> (w418:T1[])
            n304 = Spreadsheet String To Array(delimiter (Tab)=";", format string="%s", spreadsheet string=w424, array type (2D Dbl)=string[] []) -> (array=w419:string[])
            n305 = local read "_Rx Table"() -> (w417:i32)
            n306 = Delete From Array(array=w419, index=w417) -> (array with subset deleted=w421:string[])  [unwired: 1 in, 1 out]
            n307 = Delete From Array(array=w418, index=w417) -> (array with subset deleted=w428:T1[])  [unwired: 1 in, 1 out]
            n308 = property on="_Rx Table" class="MCListbox (strict)"("Val(Sgnl)"=w417) -> ()  [unwired: 2 in, 2 out]
            n309 = Array To Spreadsheet String(delimiter (Tab)=";", array=w421, 3:"%s" ("format string")) -> (spreadsheet string=w420:string)
            n310 = property on="_Control Param Array" class="Arr (strict)"("Val(Sgnl)"=w428) -> ()  [unwired: 2 in, 2 out]
            n311 = property on="Rx Signals" class="Str"("Val(Sgnl)"=w420) -> ()  [unwired: 2 in, 2 out]
            n312 = property on="_Refresh (Hidden)" class="Bool (strict)"("Val(Sgnl)"=TRUE ("Value (Signaling)")) -> ()  [unwired: 2 in, 2 out]
          }
          event "_Rx Table": Value Change {
            n313 = event-data() -> ()  [unwired: 1 in, 6 out]
            n314 = local read "Rx Signals"() -> (w440:string)
            n315 = local read "_Control Param Array"() -> (w438:T1[])
            n316 = Spreadsheet String To Array(delimiter (Tab)=";", format string="%s", spreadsheet string=w440, array type (2D Dbl)=string[] []) -> (array=w439:string[])
            n317 = local read "_Rx Table"() -> (w436:i32)
            n318 = Index Array(array=w439, index=w436) -> (element=w434:string)
            n319 = Index Array(array=w438, index=w436) -> (element=w435:T1)
            n320 = property on="_Rx Signals Mem" class="Arr (strict)"() -> ("Value"=w432:string[])  [unwired: 2 in, 2 out]
            n321 = local write "_Control Parameter"(w435) -> ()
            n322 = Search 1D Array(1D array=w432, element=w434) -> (index of element=w433:i32)  [unwired: 1 in]
            n323 = Increment(x=w433) -> (x+1=w431:i32)
            n324 = local write "_CAN Rx Signal"(w431) -> ()
            n325 = property on="_Refresh (Hidden)" class="Bool (strict)"("Val(Sgnl)"=TRUE ("Value (Signaling)")) -> ()  [unwired: 2 in, 2 out]
          }
          event "_CAN Rx Signal": Value Change {
            n326 = event-data() -> ()  [unwired: 1 in, 6 out]
            n327 = local read "_Control Param Array"() -> (w460:T1[])
            n328 = local read "Rx Signals"() -> (w454:string)
            n329 = local read "_CAN Rx Signal"() -> (w452:u16)
            n330 = local read "_Control Parameter"() -> (w461:T1)
            n331 = property on="_Rx Signals Mem" class="Arr (strict)"() -> ("Value"=w445:string[])  [unwired: 2 in, 2 out]
            n332 = Decrement(x=w452) -> (x-1=w444:u16)
            n333 = Spreadsheet String To Array(delimiter (Tab)=";", format string="%s", spreadsheet string=w454, array type (2D Dbl)=string[] []) -> (array=w453:string[])
            n334 = local read "_Rx Table"() -> (w458:i32)
            n335 = Index Array(array=w445, index=w444) -> (element=w451:string)
            n336 = Replace Array Subset(array=w453, new element=w451, index=w458) -> (w447:string[])
            n337 = Replace Array Subset(array=w460, new element=w461, index=w458) -> (w450:T1[])
            n338 = property on="_Control Param Array" class="Arr (strict)"("Val(Sgnl)"=w450) -> ()  [unwired: 2 in, 2 out]
            n339 = Array To Spreadsheet String(delimiter (Tab)=";", array=w447, 3:"%s" ("format string")) -> (spreadsheet string=w446:string)
            n340 = property on="Rx Signals" class="Str"("Val(Sgnl)"=w446) -> ()  [unwired: 2 in, 2 out]
            n341 = property on="_Refresh (Hidden)" class="Bool (strict)"("Val(Sgnl)"=TRUE ("Value (Signaling)")) -> ()  [unwired: 2 in, 2 out]
          }
          event "_Tx.Up": Value Change {
            n342 = event-data() -> ()  [unwired: 1 in, 6 out]
            n343 = local write "_Tx.Up"(FALSE ("_Up")) -> ()
            n344 = local read "Tx Signals"() -> (w471:string)
            n345 = property on="_Tx Table" class="MCListbox (strict)"() -> ("ItemNames"=w463:string[][])  [unwired: 2 in, 2 out]
            n346 = local read "CalPointIDs"() -> (w477:sgl[])
            n347 = local read "_Tx Table"() -> (w462:i32)
            n348 = Array Size(array=w463) -> (size(s)=w483:i32[])
            n349 = Index Array(array=w483) -> (element=w484:i32)  [unwired: 1 in]
            n350 = Spreadsheet String To Array(delimiter (Tab)=";", format string="%s", spreadsheet string=w471, array type (2D Dbl)=string[] []) -> (array=w470:string[])
            n351 = Decrement(x=w484) -> (x-1=w481:i32)
            n352 = Decrement(x=w462) -> (x-1=w482:i32)
            n353 = Delete From Array(array=w470, index=w462) -> (deleted portion=w476:string, array with subset deleted=w478:string[])  [unwired: 1 in]
            n354 = Delete From Array(array=w477, index=w462) -> (deleted portion=w475:sgl, array with subset deleted=w479:sgl[])  [unwired: 1 in]
            n355 = In Range and Coerce(upper limit=w481, x=w482, lower limit=0) -> (coerced(x)=w466:i32)  [unwired: 1 out]
            n356 = Insert Into Array(array=w478, index=w466, new element=w476) -> (w467:string[])
            n357 = Insert Into Array(array=w479, index=w466, new element=w475) -> (w464:sgl[])
            n358 = property on="CalPointIDs" class="Arr (strict)"("Val(Sgnl)"=w464) -> ()  [unwired: 2 in, 2 out]
            n359 = Array To Spreadsheet String(delimiter (Tab)=";", array=w467, 3:"%s" ("format string")) -> (spreadsheet string=w465:string)
            n360 = local write "_Tx Table"(w466) -> ()
            n361 = property on="Tx Signals" class="Str"("Val(Sgnl)"=w465) -> ()  [unwired: 2 in, 2 out]
            n362 = property on="_Refresh (Hidden)" class="Bool (strict)"("Val(Sgnl)"=TRUE ("Value (Signaling)")) -> ()  [unwired: 2 in, 2 out]
          }
          event "_Tx.Down": Value Change {
            n363 = event-data() -> ()  [unwired: 1 in, 6 out]
            n364 = local write "_Tx.Down"(FALSE ("_Up")) -> ()
            n365 = local read "Tx Signals"() -> (w496:string)
            n366 = property on="_Tx Table" class="MCListbox (strict)"() -> ("ItemNames"=w488:string[][])  [unwired: 2 in, 2 out]
            n367 = local read "CalPointIDs"() -> (w502:sgl[])
            n368 = local read "_Tx Table"() -> (w487:i32)
            n369 = Array Size(array=w488) -> (size(s)=w508:i32[])
            n370 = Index Array(array=w508) -> (element=w509:i32)  [unwired: 1 in]
            n371 = Spreadsheet String To Array(delimiter (Tab)=";", format string="%s", spreadsheet string=w496, array type (2D Dbl)=string[] []) -> (array=w495:string[])
            n372 = Decrement(x=w509) -> (x-1=w506:i32)
            n373 = Increment(x=w487) -> (x+1=w507:i32)
            n374 = Delete From Array(array=w495, index=w487) -> (deleted portion=w501:string, array with subset deleted=w503:string[])  [unwired: 1 in]
            n375 = Delete From Array(array=w502, index=w487) -> (deleted portion=w500:sgl, array with subset deleted=w504:sgl[])  [unwired: 1 in]
            n376 = In Range and Coerce(upper limit=w506, x=w507, lower limit=0) -> (coerced(x)=w491:i32)  [unwired: 1 out]
            n377 = Insert Into Array(array=w503, index=w491, new element=w501) -> (w492:string[])
            n378 = Insert Into Array(array=w504, index=w491, new element=w500) -> (w489:sgl[])
            n379 = property on="CalPointIDs" class="Arr (strict)"("Val(Sgnl)"=w489) -> ()  [unwired: 2 in, 2 out]
            n380 = Array To Spreadsheet String(delimiter (Tab)=";", array=w492, 3:"%s" ("format string")) -> (spreadsheet string=w490:string)
            n381 = local write "_Tx Table"(w491) -> ()
            n382 = property on="Tx Signals" class="Str"("Val(Sgnl)"=w490) -> ()  [unwired: 2 in, 2 out]
            n383 = property on="_Refresh (Hidden)" class="Bool (strict)"("Val(Sgnl)"=TRUE ("Value (Signaling)")) -> ()  [unwired: 2 in, 2 out]
          }
          event "_Tx.Insert": Value Change {
            n384 = event-data() -> ()  [unwired: 1 in, 6 out]
            n385 = local write "_Tx.Insert"(FALSE ("_Up")) -> ()
            n386 = local read "Tx Signals"() -> (w525:string)
            n387 = local read "CalPointIDs"() -> (w519:sgl[])
            n388 = local read "_CAN Tx Signal"() -> (w517:u16)
            n389 = local read "_Tx Table"() -> (w529:i32)
            n390 = Spreadsheet String To Array(delimiter (Tab)=";", format string="%s", spreadsheet string=w525, array type (2D Dbl)=string[] []) -> (array=w518:string[])
            n391 = local read "_CalPoints Select"() -> (w513:u32)
            n392 = Decrement(x=w517) -> (x-1=w514:u16)
            n393 = property on="_Tx Signals Mem" class="Arr (strict)"() -> ("Value"=w512:string[])  [unwired: 2 in, 2 out]
            n394 = Index Array(array=w512, index=w514) -> (element=w516:string)
            n395 = Increment(x=w529) -> (x+1=w515:i32)
            n396 = Insert Into Array(array=w518, index=w515, new element=w516) -> (w522:string[])
            n397 = Insert Into Array(array=w519, index=w515, new element=w513) -> (w520:sgl[])
            n398 = property on="_Tx Table" class="MCListbox (strict)"("Val(Sgnl)"=w515) -> ()  [unwired: 2 in, 2 out]
            n399 = property on="CalPointIDs" class="Arr (strict)"("Val(Sgnl)"=w520) -> ()  [unwired: 2 in, 2 out]
            n400 = Array To Spreadsheet String(delimiter (Tab)=";", array=w522, 3:"%s" ("format string")) -> (spreadsheet string=w521:string)
            n401 = property on="Tx Signals" class="Str"("Val(Sgnl)"=w521) -> ()  [unwired: 2 in, 2 out]
            n402 = property on="_Refresh (Hidden)" class="Bool (strict)"("Val(Sgnl)"=TRUE ("Value (Signaling)")) -> ()  [unwired: 2 in, 2 out]
          }
          event "_Tx.Delete": Value Change {
            n403 = event-data() -> ()  [unwired: 1 in, 6 out]
            n404 = local write "_Tx.Delete"(FALSE ("_Up")) -> ()
            n405 = local read "Tx Signals"() -> (w539:string)
            n406 = local read "CalPointIDs"() -> (w543:sgl[])
            n407 = local read "_Tx Table"() -> (w532:i32)
            n408 = Spreadsheet String To Array(delimiter (Tab)=";", format string="%s", spreadsheet string=w539, array type (2D Dbl)=string[] []) -> (array=w538:string[])
            n409 = Delete From Array(array=w538, index=w532) -> (array with subset deleted=w534:string[])  [unwired: 1 in, 1 out]
            n410 = Delete From Array(array=w543, index=w532) -> (array with subset deleted=w533:sgl[])  [unwired: 1 in, 1 out]
            n411 = property on="_Tx Table" class="MCListbox (strict)"("Val(Sgnl)"=w532) -> ()  [unwired: 2 in, 2 out]
            n412 = property on="CalPointIDs" class="Arr (strict)"("Val(Sgnl)"=w533) -> ()  [unwired: 2 in, 2 out]
            n413 = Array To Spreadsheet String(delimiter (Tab)=";", array=w534, 3:"%s" ("format string")) -> (spreadsheet string=w535:string)
            n414 = property on="Tx Signals" class="Str"("Val(Sgnl)"=w535) -> ()  [unwired: 2 in, 2 out]
            n415 = property on="_Refresh (Hidden)" class="Bool (strict)"("Val(Sgnl)"=TRUE ("Value (Signaling)")) -> ()  [unwired: 2 in, 2 out]
          }
          event "_Tx Table": Value Change {
            n416 = event-data() -> ()  [unwired: 1 in, 6 out]
            n417 = local read "Tx Signals"() -> (w555:string)
            n418 = local read "CalPointIDs"() -> (w553:sgl[])
            n419 = Spreadsheet String To Array(delimiter (Tab)=";", format string="%s", spreadsheet string=w555, array type (2D Dbl)=string[] []) -> (array=w554:string[])
            n420 = local read "_Tx Table"() -> (w552:i32)
            n421 = Index Array(array=w554, index=w552) -> (element=w550:string)
            n422 = Index Array(array=w553, index=w552) -> (element=w551:sgl)
            n423 = property on="_Tx Signals Mem" class="Arr (strict)"() -> ("Value"=w546:string[])  [unwired: 2 in, 2 out]
            n424 = Search 1D Array(1D array=w546, element=w550) -> (index of element=w549:i32)  [unwired: 1 in]
            n425 = local write "_CalPoints Select"(w551) -> ()
            n426 = Increment(x=w549) -> (x+1=w547:i32)
            n427 = local write "_CAN Tx Signal"(w547) -> ()
            n428 = property on="_Refresh (Hidden)" class="Bool (strict)"("Val(Sgnl)"=TRUE ("Value (Signaling)")) -> ()  [unwired: 2 in, 2 out]
          }
          event "_CalPoints Select", "_CAN Tx Signal": Value Change {
            n429 = event-data() -> ()  [unwired: 1 in, 6 out]
            n430 = local read "Tx Signals"() -> (w570:string)
            n431 = local read "CalPointIDs"() -> (w575:sgl[])
            n432 = local read "_CAN Tx Signal"() -> (w568:u16)
            n433 = property on="_Tx Signals Mem" class="Arr (strict)"() -> ("Value"=w560:string[])  [unwired: 2 in, 2 out]
            n434 = Decrement(x=w568) -> (x-1=w561:u16)
            n435 = Spreadsheet String To Array(delimiter (Tab)=";", format string="%s", spreadsheet string=w570, array type (2D Dbl)=string[] []) -> (array=w569:string[])
            n436 = local read "_Tx Table"() -> (w574:i32)
            n437 = Index Array(array=w560, index=w561) -> (element=w567:string)
            n438 = Replace Array Subset(array=w569, new element=w567, index=w574) -> (w564:string[])
            n439 = Replace Array Subset(array=w575, new element="_CalPoints Select", index=w574) -> (w563:sgl[])
            n440 = property on="CalPointIDs" class="Arr (strict)"("Val(Sgnl)"=w563) -> ()  [unwired: 2 in, 2 out]
            n441 = Array To Spreadsheet String(delimiter (Tab)=";", array=w564, 3:"%s" ("format string")) -> (spreadsheet string=w562:string)
            n442 = property on="Tx Signals" class="Str"("Val(Sgnl)"=w562) -> ()  [unwired: 2 in, 2 out]
            n443 = property on="_Refresh (Hidden)" class="Bool (strict)"("Val(Sgnl)"=TRUE ("Value (Signaling)")) -> ()  [unwired: 2 in, 2 out]
          }
          event "_CAN Interface", "_Control Param Array", "CalPointIDs": Value Change {
            n444 = event-data() -> ()  [unwired: 1 in, 6 out]
            n445 = local read "_Control Param Array"() -> (w581:T1[])
            n446 = local read "_CAN Interface"() -> (w582:u8)
            n447 = Array To Spreadsheet String(delimiter (Tab)=",", array=w581, 3:"%d" ("format string")) -> (spreadsheet string=w578:string)
            n448 = property on="CAN Interface" class="DigNum (strict)"("Val(Sgnl)"=w582) -> ()  [unwired: 2 in, 2 out]
            n449 = property on="ControlParamMem" class="Str"("Val(Sgnl)"=w578) -> ()  [unwired: 2 in, 2 out]
            n450 = property on="_Refresh (Hidden)" class="Bool (strict)"("Val(Sgnl)"=TRUE ("Value (Signaling)")) -> ()  [unwired: 2 in, 2 out]
          }
          event "CAN_Run": Value Change {
            n451 = event-data() -> ()  [unwired: 1 in, 6 out]
            n452 = local read "CAN_Run"() -> (w584:bool)
            n453 = Select(t=T3."Disabled and Grayed Out" ("Disabled"), s=w584, f=T3."Enabled" ("Disabled")) -> (s? t:f=w583:T3)
            n454 = property on="_Rx.Insert" class="Bool (strict)"("DisabledEnum"=w583) -> ()  [unwired: 2 in, 2 out]
            n455 = property on="_Rx.Delete" class="Bool (strict)"("DisabledEnum"=w583) -> ()  [unwired: 2 in, 2 out]
            n456 = property on="_Rx.Up" class="Bool (strict)"("DisabledEnum"=w583) -> ()  [unwired: 2 in, 2 out]
            n457 = property on="_Rx.Down" class="Bool (strict)"("DisabledEnum"=w583) -> ()  [unwired: 2 in, 2 out]
            n458 = property on="_Tx.Insert" class="Bool (strict)"("DisabledEnum"=w583) -> ()  [unwired: 2 in, 2 out]
            n459 = property on="_Tx.Delete" class="Bool (strict)"("DisabledEnum"=w583) -> ()  [unwired: 2 in, 2 out]
            n460 = property on="_Tx.Up" class="Bool (strict)"("DisabledEnum"=w583) -> ()  [unwired: 2 in, 2 out]
            n461 = property on="_Tx.Down" class="Bool (strict)"("DisabledEnum"=w583) -> ()  [unwired: 2 in, 2 out]
            n462 = property on="_CAN Rx Signal" class="Ring (strict)"("DisabledEnum"=w583) -> ()  [unwired: 2 in, 2 out]
            n463 = property on="_CAN Tx Signal" class="Ring (strict)"("DisabledEnum"=w583) -> ()  [unwired: 2 in, 2 out]
            n464 = property on="_Control Parameter" class="Enum (strict)"("DisabledEnum"=w583) -> ()  [unwired: 2 in, 2 out]
            n465 = property on="Deployed Databases" class="LstBox (strict)"("DisabledEnum"=w583) -> ()  [unwired: 2 in, 2 out]
            n466 = property on="Deployed Clusters" class="LstBox (strict)"("DisabledEnum"=w583) -> ()  [unwired: 2 in, 2 out]
            n467 = property on="Deployed ECUs" class="LstBox (strict)"("DisabledEnum"=w583) -> ()  [unwired: 2 in, 2 out]
            n468 = property on="_CAN Interface" class="Ring (strict)"("DisabledEnum"=w583) -> ()  [unwired: 2 in, 2 out]
            n469 = property on="Baud_Rate" class="DigNum (strict)"("DisabledEnum"=w583) -> ()  [unwired: 2 in, 2 out]
            n470 = property on="Intf_CAN_Term" class="Bool (strict)"("DisabledEnum"=w583) -> ()  [unwired: 2 in, 2 out]
            n471 = property on="_CalPoints Select" class="Ring (strict)"("DisabledEnum"=w583) -> ()  [unwired: 2 in, 2 out]
            n472 = property on="Refresh Database" class="Bool (strict)"("DisabledEnum"=w583) -> ()  [unwired: 2 in, 2 out]
          }
          event "Deployed Databases", "Deployed Clusters", "Deployed ECUs": Value Change {
            n473 = event-data() -> ()  [unwired: 1 in, 6 out]
            n474 = property on="_Refresh (Hidden)" class="Bool (strict)"("Val(Sgnl)"=TRUE ("Value (Signaling)")) -> ()  [unwired: 2 in, 2 out]
          }
        }
        n475 = local read "XNET_Fault"() -> (w168:bool)
        n476 = call "ChangeIndicator.vi"("Input"=w168) -> ("Change"=w172:bool)  [unwired: 9 in]
        n477 = call "ChangeIndicator.vi"("Input"=w167) -> ("Change"=w171:bool)  [unwired: 9 in]
        n478 = call "ChangeIndicator.vi"("Input"=w166) -> ("Change"=w170:bool)  [unwired: 9 in]
        n479 = Compound Arithmetic op=OR(w172, w171, w170) -> (w169:bool)
        n480 = case shown="True" w169 {
          tunnel: w168 -> [_ w185]
          tunnel: w167 -> [_ w184]
          tunnel: w166 -> [_ w183]
          frame False {
          }
          frame True {
            n481 = Bundle By Name(cluster=T4 {"Status"=FALSE, "Code"=0, "Desc"="dsfsasd"} ("XNET Error"), "Status"=w185, "Code"=w184, "Desc"=w183) -> (w179:T4)
            n482 = call <vilib>:"Simple Error Handler.vi"("type of dialog (OK msg:1)"=u16 0, "error in (no error)"=w179) -> ("message"=w181:string)  [unwired: 3 in, 4 out]
            n483 = Bundle By Name(cluster=w179, "Desc"=w181) -> (→"_XNET Error":T4)
          }
        }
        n484 = local read "DatabaseAlias"() -> (w175:string)
        n485 = call "ChangeIndicator.vi"("Input"=w175) -> ("Change"=w174:bool)  [unwired: 9 in]
        n486 = case shown="True" w174 {
          tunnel: w175 -> [_ w189]
          tunnel: "------ No Database Selected ------" ("DatabaseAlias") -> [_ w186]
          frame False {
          }
          frame True {
            n487 = Spreadsheet String To Array(format string="%s", spreadsheet string=w189, array type (2D Dbl)=string[] []) -> (array=w188:string[])  [unwired: 1 in]
            n488 = Build Array (concatenate)(w186, w188) -> (w187:string[])
            n489 = property on="Deployed Databases" class="LstBox (strict)"("Item Names"=w187) -> ()  [unwired: 2 in, 2 out]
          }
        }
      }
    }
  }
